vi "eyecat v01 Mc 804 ROB_JS.vi"() -> ()   [LabVIEW 2014]
doc: "This VI is an upgrade from the WIN 1_v4 that implements the ageing subrutine"
uses:
  <vilib>/Utility/file.llb/Write To Spreadsheet File (string).vi
  <vilib>/Utility/file.llb/Read From Spreadsheet File (string).vi
  <vilib>/regexp/Match Regular Expression.xnode
  Controls Win/Control 3.ctl
  <vilib>/Utility/miscctls.llb/LVRowAndColumnTypeDef.ctl
  <vilib>/Platform/TimedLoop/XDataNode/XDataNode.xnode
  <vilib>/Platform/TimedLoop/XDataNode/nitl_modes.ctl
  <vilib>/Platform/TimedLoop/XDataNode/XDNodeRunTimeDep.lvlib
  <vilib>/Platform/TimedLoop/XDataNode/wakeup.ctl
  <vilib>/Platform/TimedLoop/XDataNode/timing_clust.ctl
  Buttons/Numeric control.ctl
  Buttons/String input.ctl
  Buttons/Numeric indicator.ctl
  Buttons/String output.ctl
panel:
  out "MKS 1":i16
  out "MKS 2":i16
  out "output cluster":T2
  out "Full system?":bool
  out "Log interval (seconds)":T1
  in  "Flow rate Age":dbl
  in  "Inlet temp Age":dbl
  out "Stopped?":bool
  in  "Stop Cmd":T1
  out "Connected?":bool
  out "Error":dbl
  out "Iteration Duration":i64
  out "Finished Late? [i-1]":bool
  in  "SO2 ppm":dbl
  out "Furnace temp 1":dbl
  out "stop 2":bool
  in  "Enum 1":i16=1
  in  "Acknowledge":bool
  out "Test number":u16
  out "Flag1":bool=TRUE
  out "EditPos Subc":T3
  out "Flag 2":bool=TRUE
  in  "Tab Control":T4(tab)
  out "Doors Unlocked":bool
  in  "Temperature Limit (°C)":T1=800.0 min=0.0 max=1200.0 step=1.0
  in  "Log Test Button":bool
  in  "File Name":T5
  in  "File Path":path=path "C:/DATA LOG"
  out "Fail":bool
  out "Pass":bool
  in  "Select Test Type":T6(radio)
  out "Standby":bool
  out "Doors Open":bool
  out "Extractor Fan On":bool
  out "Test In Progress":bool
  out "Cool Down":bool
  out "System Alarm":bool
  in  "Execute Leak Test Button":bool
  in  "Stop Test Button":bool
  in  "Start Test Button":bool
  in  "Advanced settings":bool
  out "Lambda 1":dbl
  out "FlowRate":dbl
  out "Tank P":dbl
  out "O2 Rapidox":dbl
  in  "AirB":dbl
  in  "H2O":dbl
  in  "SO2":dbl
  in  "N2":dbl
  in  "CO2":dbl
  in  "NO":dbl
  in  "Air":dbl
  in  "HC":dbl
  in  "CO":dbl
  in  "Output range Lo":dbl=20.0
  in  "Output range Hi":dbl=200.0
  in  "Lambda D":dbl
  in  "Lambda I":dbl
  in  "Lambda P":dbl
  in  "Tank Lo":dbl=7.0
  in  "Tank Hi":dbl=8.0
  in  "Furnace lambda":dbl
  in  "Air Bal Factor":dbl
  in  "Air open loop factor":dbl
  in  "Lambda Setpoint":dbl=1.08
  in  "N2 Age":dbl
  in  "Bed target":dbl=750.0
  in  "Furnace SP WarmUp":dbl=1000.0
  in  "HC Inj Control":dbl
  in  "HC Bal Factor":dbl
  in  "HC Cyc Factor":dbl
  in  "Fan Speed V":dbl
  in  "Air O2 Rap limit":dbl
  in  "Factor Air Baseline":dbl
  in  "SW time":dbl
  in  "Inlet Temperature (°C)":T1=400.0 min=350.0 max=1000.0 step=1.0
  in  "Inlet LAMBDA Rich":T1=0.9 min=0.85 max=0.96 step=0.001
  in  "Inlet LAMBDA Lean":T1=1.2 min=1.02 max=3.0 step=0.001
  in  "Test Stop temperature (°C)":T1=300.0 min=100.0 max=1000.0 step=1.0
  in  "Test Start Temperature (°C)":T1=125.0 min=0.0 max=500.0 step=1.0
  in  "Furnace Ramp Rate (°C/min)":T1=15.0 min=1.0 max=50.0 step=0.1
  in  "NO:CO Ratio":T1=1.1 min=1.0 max=5.0 step=0.1
  in  "Inlet O2 (%)":T1=0.5 min=0.0 max=14.0 step=0.01
  in  "Inlet LAMBDA":T1=1.0 min=0.6 max=3.0 step=0.001
  out "Space Velocity (h-1)":T7
  out "Vol Flow @ STP (l/min)":T7
  in  "Test Flow Rate(g/s)":T1 min=0.0 max=100.0 step=0.01
  out "Sample Volume (litres)":T7
  in  "Number of Samples":T1=1.0 min=1.0 max=6.0 step=1.0
  in  "Sample Diameter (mm)":T1
  out "CO Theory (%)":T7 format="%#_3g"
  out "CO Theory (%)":T7 format="%#_3g"
  out "HC Theory (%)":T7
  in  "Sample Length (mm)":T1 min=0.0 step=0.5
  in  "NO ppm SW":dbl=500.0 caption="NO (ppm)" min=0.0 max=500.0 step=1.0
  in  "NO ppm Loff":T1 caption="NO ppm"
  out "Inlet Temp":dbl
  in  "Delete sCycle":bool
  in  "Load sCycle":bool
  in  "Save sCycle":bool
  in  "Clear subcycle":bool
  in  "Clear Cycle Pattern":bool
  in  "Save Cycle":bool
  in  "Load Cycle":bool
  in  "Delete Cycle":bool
  out "Test Compiled":bool
  in  "Compile Test Button":bool
  in  "Sub-Cycle List":i32(listbox)=1
  in  "Cycle List":i32(listbox)=2
  out "Total Test Duration (hrs)":T8
  in  "Ageing Gas":enum32{"Radio Selection 1", "Radio Selection 2"}(radio)
  in  "Sub-Cycle Pattern":string[][](table) caption="Subcycle pattern"
  in  "Total Number of Cycles":T1=1.0 min=1.0 max=10000.0 step=1.0
  in  "Cycle Pattern":string[][](table)
  in  "Sub-Cycle Name":T5
  in  "Cycle Name":T5
  out "Heat Exchanger Temperatures (°C)":dynamicdata(graph)
  out "Flow Rate (g/s)":dynamicdata(graph)
  out "Sample Temperatures (°C)":dynamicdata(graph)
  out "System Temperatures (°C)":dynamicdata(graph)
  out "HC Concentration (ppm)":dynamicdata(graph)
  out "Lambda":dynamicdata(graph)
  out "M584L Upstream & Downstream":dynamicdata(graph)
  out "NO Concentration (ppm)":dynamicdata(graph)
  in  "Purge System":bool
  in  "Alarm ack":bool
  in  "Clear log":bool
  out "Table":string[][](table)
  out "Soft Alarm":bool
  out "Hard Alarm":bool
  # "Test Type"
  # "Test Commands"
  # "System Indicators"
  # "Leak Test"
  # "Catalyst Specification"
  # "Lightoff Settings"
  # "Furnace Lightoff Settings"
  # "Sweep Settings"
  # "CO/HC Lightoff Settings"
  # "0.96 < lambda < 0.85"
  # "1.02< lambda < 1.6"
  # "350 < Tinlet < 1000"
  # "NO Lightoff Settings"
  # "Flow Specification"
  # "Cycle Compiled"
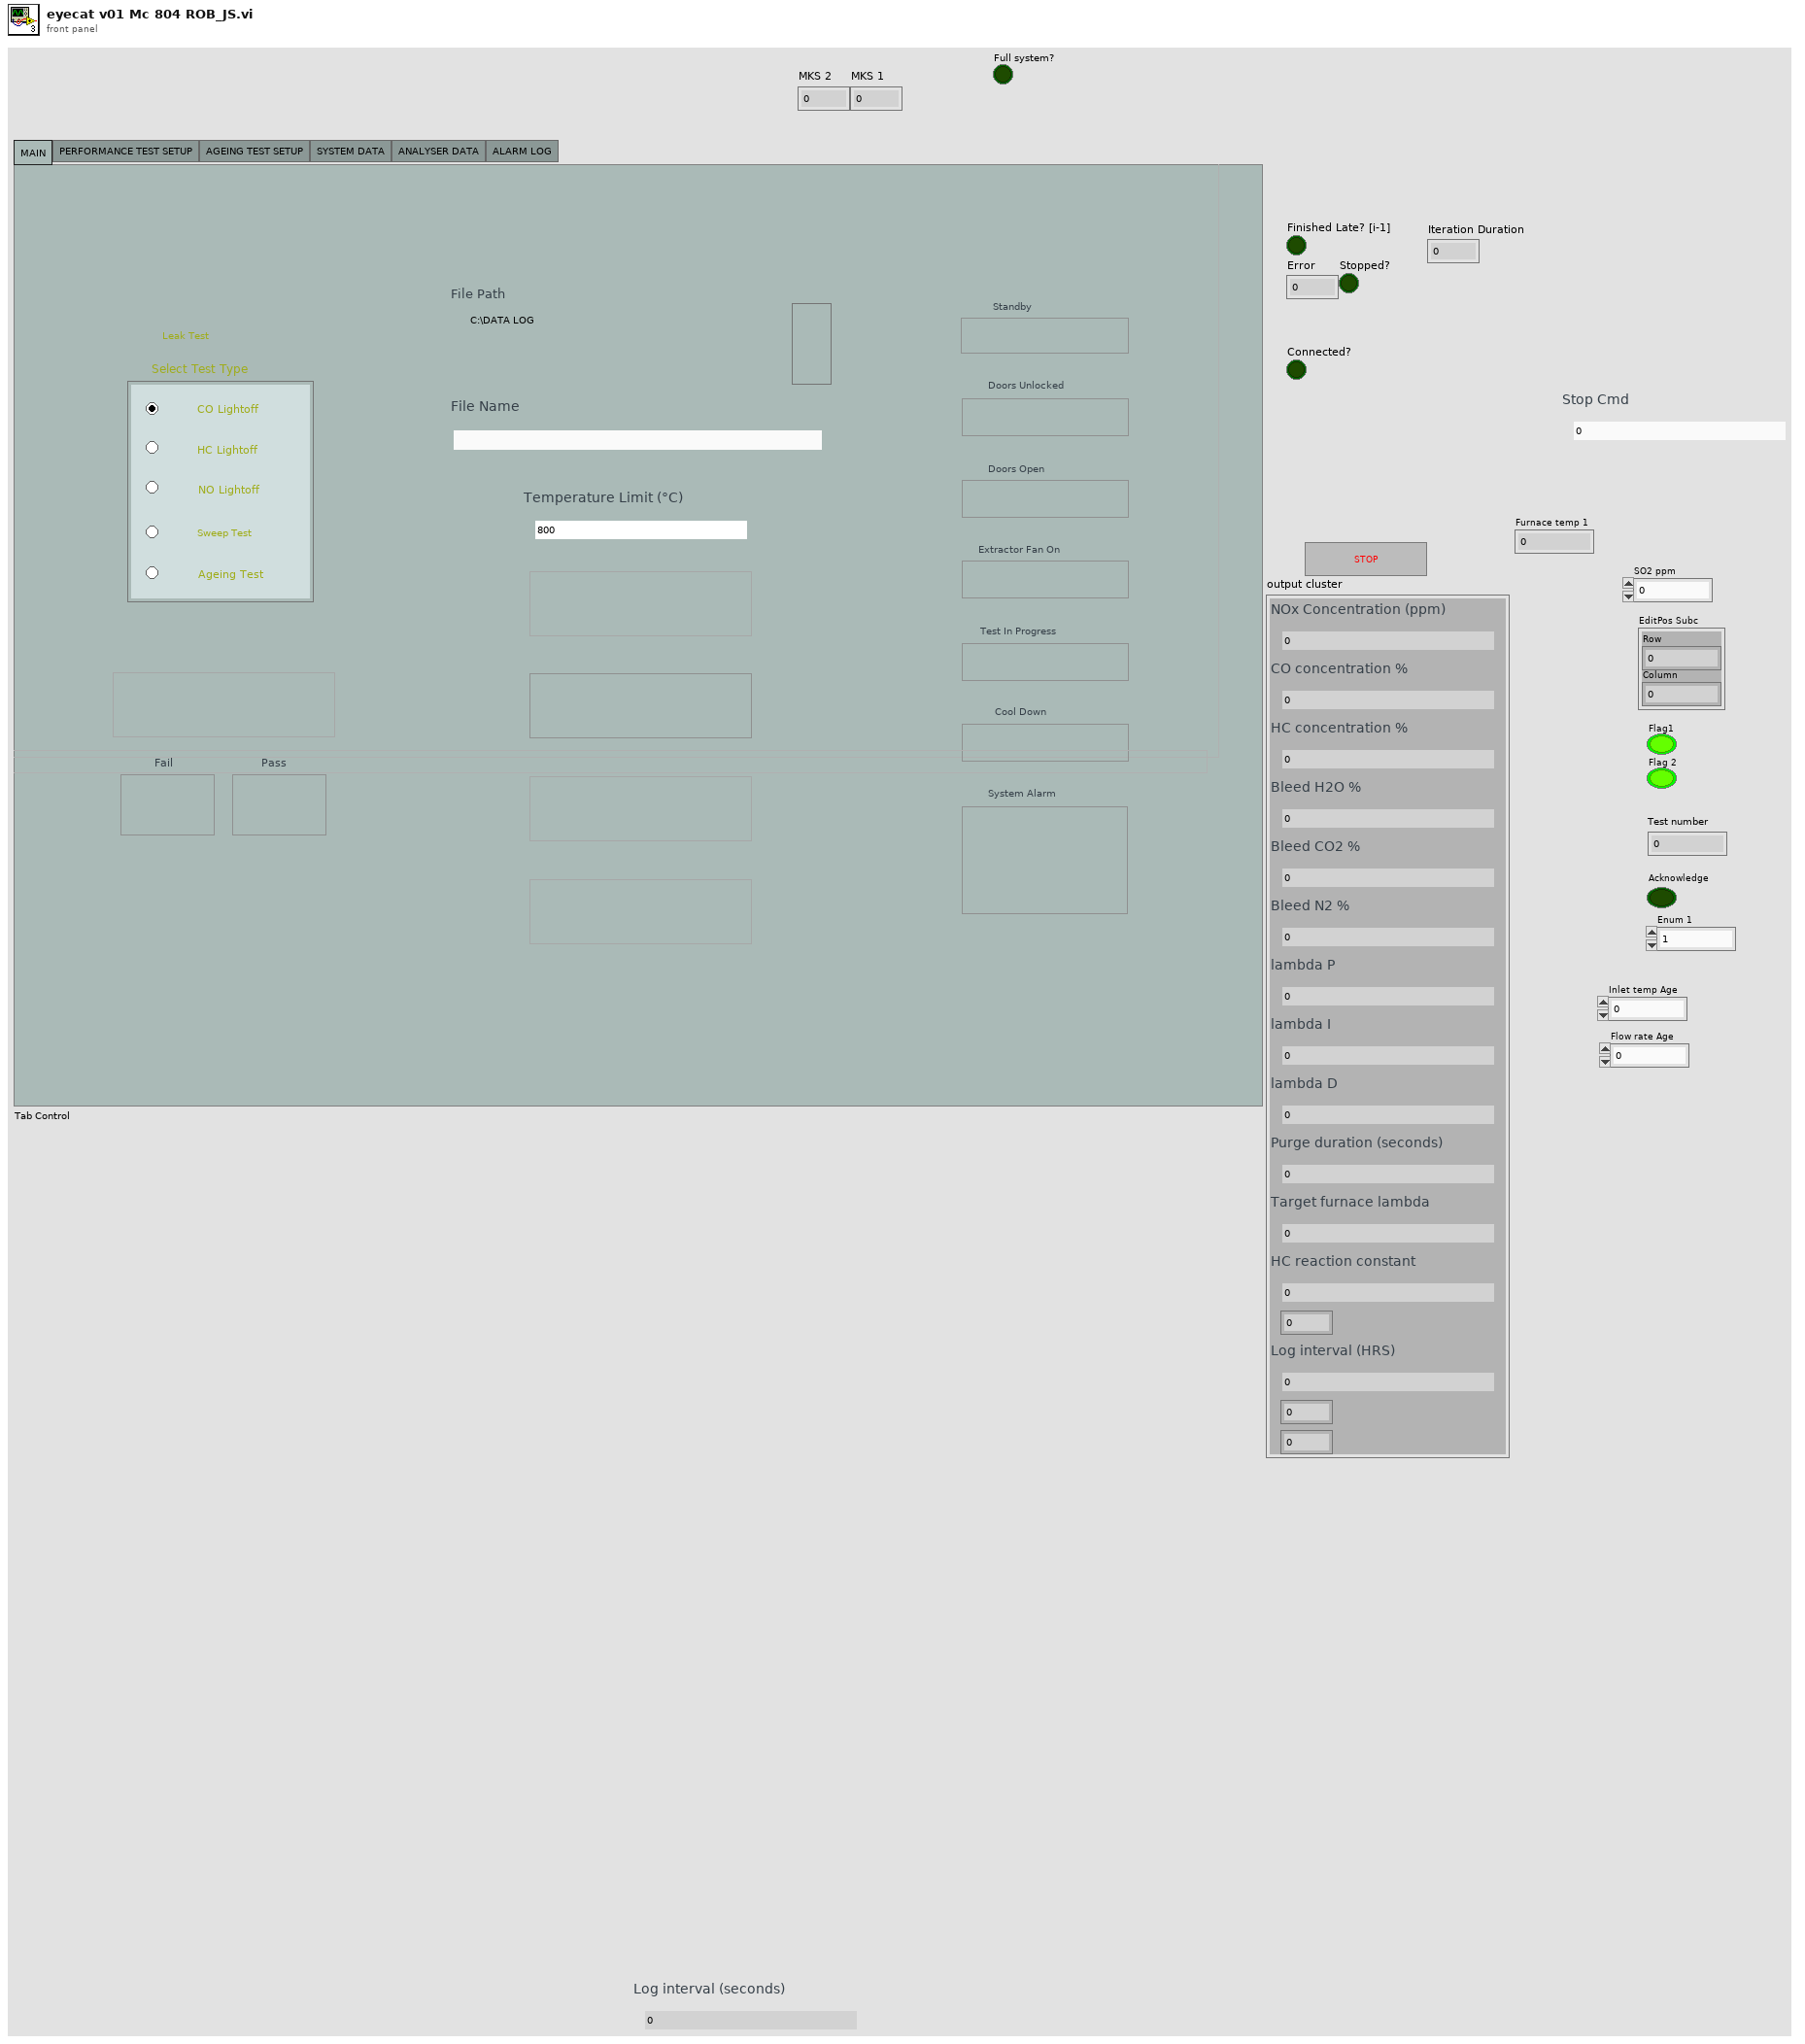
[diagram p1: front panel]
types:
  T1 = typedef "Numeric control.ctl" = dbl
  T2 = cluster{"NOx Concentration (ppm)":T1, "CO concentration %":T1, "HC concentration %":T1, "Bleed H2O %":T1, "Bleed CO2 %":T1, "Bleed N2 %":T1, "lambda P":T1, "lambda I":T1, "lambda D":T1, "Purge duration (seconds)":T1, "Target furnace lambda":T1, "HC reaction constant":T1, i16, "Log interval (HRS)":T1, i16, i16}
  T3 = typedef "LVRowAndColumnTypeDef.ctl" = cluster{"Row":i32, "Column":i32}
  T4 = enum32{"MAIN", "PERFORMANCE TEST SETUP", "AGEING TEST SETUP", "SYSTEM DATA", "ANALYSER DATA", "ALARM LOG"}
  T5 = typedef "String input.ctl" = string
  T6 = enum32{"CO Lightoff", "HC Lightoff", "NO Lightoff", "Sweep Test", "Ageing Test"}
  T7 = typedef "Numeric indicator.ctl" = dbl
  T8 = typedef "String output.ctl" = string
  T9 = typedef "XDNodeRunTimeDep.lvlib/nitl_modes.ctl" = enum32{"No Change", "Process missed periods, maintain original phase", "Discard missed periods, maintain original phase", "Process missed periods, ignore original phase", "Discard missed periods, ignore original phase"}
  T10 = typedef "Control 3.ctl" = enum16{"main", "start test", "save subc", "load subc", "delete subc", "clear table 1", "update list 1", "save cycle", "load cycle", "delete cycle", "clear table 2", "update list 2", "calc HC CO", "Total time calc", "update Cycle pattern ", "load cycle name", "convert to num", "load test array", "check scycle name", "check cycle name", "Multigas connect", "Multigas disconnect"}
  T11 = typedef "XDNodeRunTimeDep.lvlib/timing_clust.ctl" = cluster{"Expected End [f-1]":u64, "Actual End [f-1]":u64, "Finished Late? [f-1]":bool, "Expected End [i-1]":u64, "Actual End [i-1]":u64, "Finished Late? [i-1]":bool, "Expected Start [i]":u64, "Actual Start [i]":u64, "Expected Start [f]":u64, "Actual Start [f]":u64, "Source Name":string, "Structure Name":string, "Period":i64, "Deadline":i64, "Offset":i64, "Start":i64, "Priority":i32, "Timeout":i32, "Mode":T9, "Wakeup Reason":T12, "Error":errorcluster, "Source Type":string, "Secondary Source Type":string, "Global End Time":u64, "Global Start Time":u64, "Frame Duration":u64, "Iteration Duration":u64, "Assigned CPU":i32, "I/O Scan Engine Mode":u32}
  T12 = typedef "XDNodeRunTimeDep.lvlib/wakeup.ctl" = enum32{"Normal", "Aborted", "Asynchronous wakeup", "Timing source error", "Timed loop error", "Timeout"}
  T13 = enum8{"Enabled", "Disabled", "Disabled and Grayed Out"}
  T14 = cluster{"NOx Concentration (ppm)":T1, "CO concentration %":T1, "HC concentration %":T1, "Bleed H2O %":T1, "Bleed CO2 %":T1, "Bleed N2 %":T1, "lambda P":T1, "lambda I":T1, "lambda D":T1, "Purge duration (seconds)":T1, "Target furnace lambda":T1, "HC reaction constant":T1, "Full System?":i16, "Log interval (HRS)":T1}
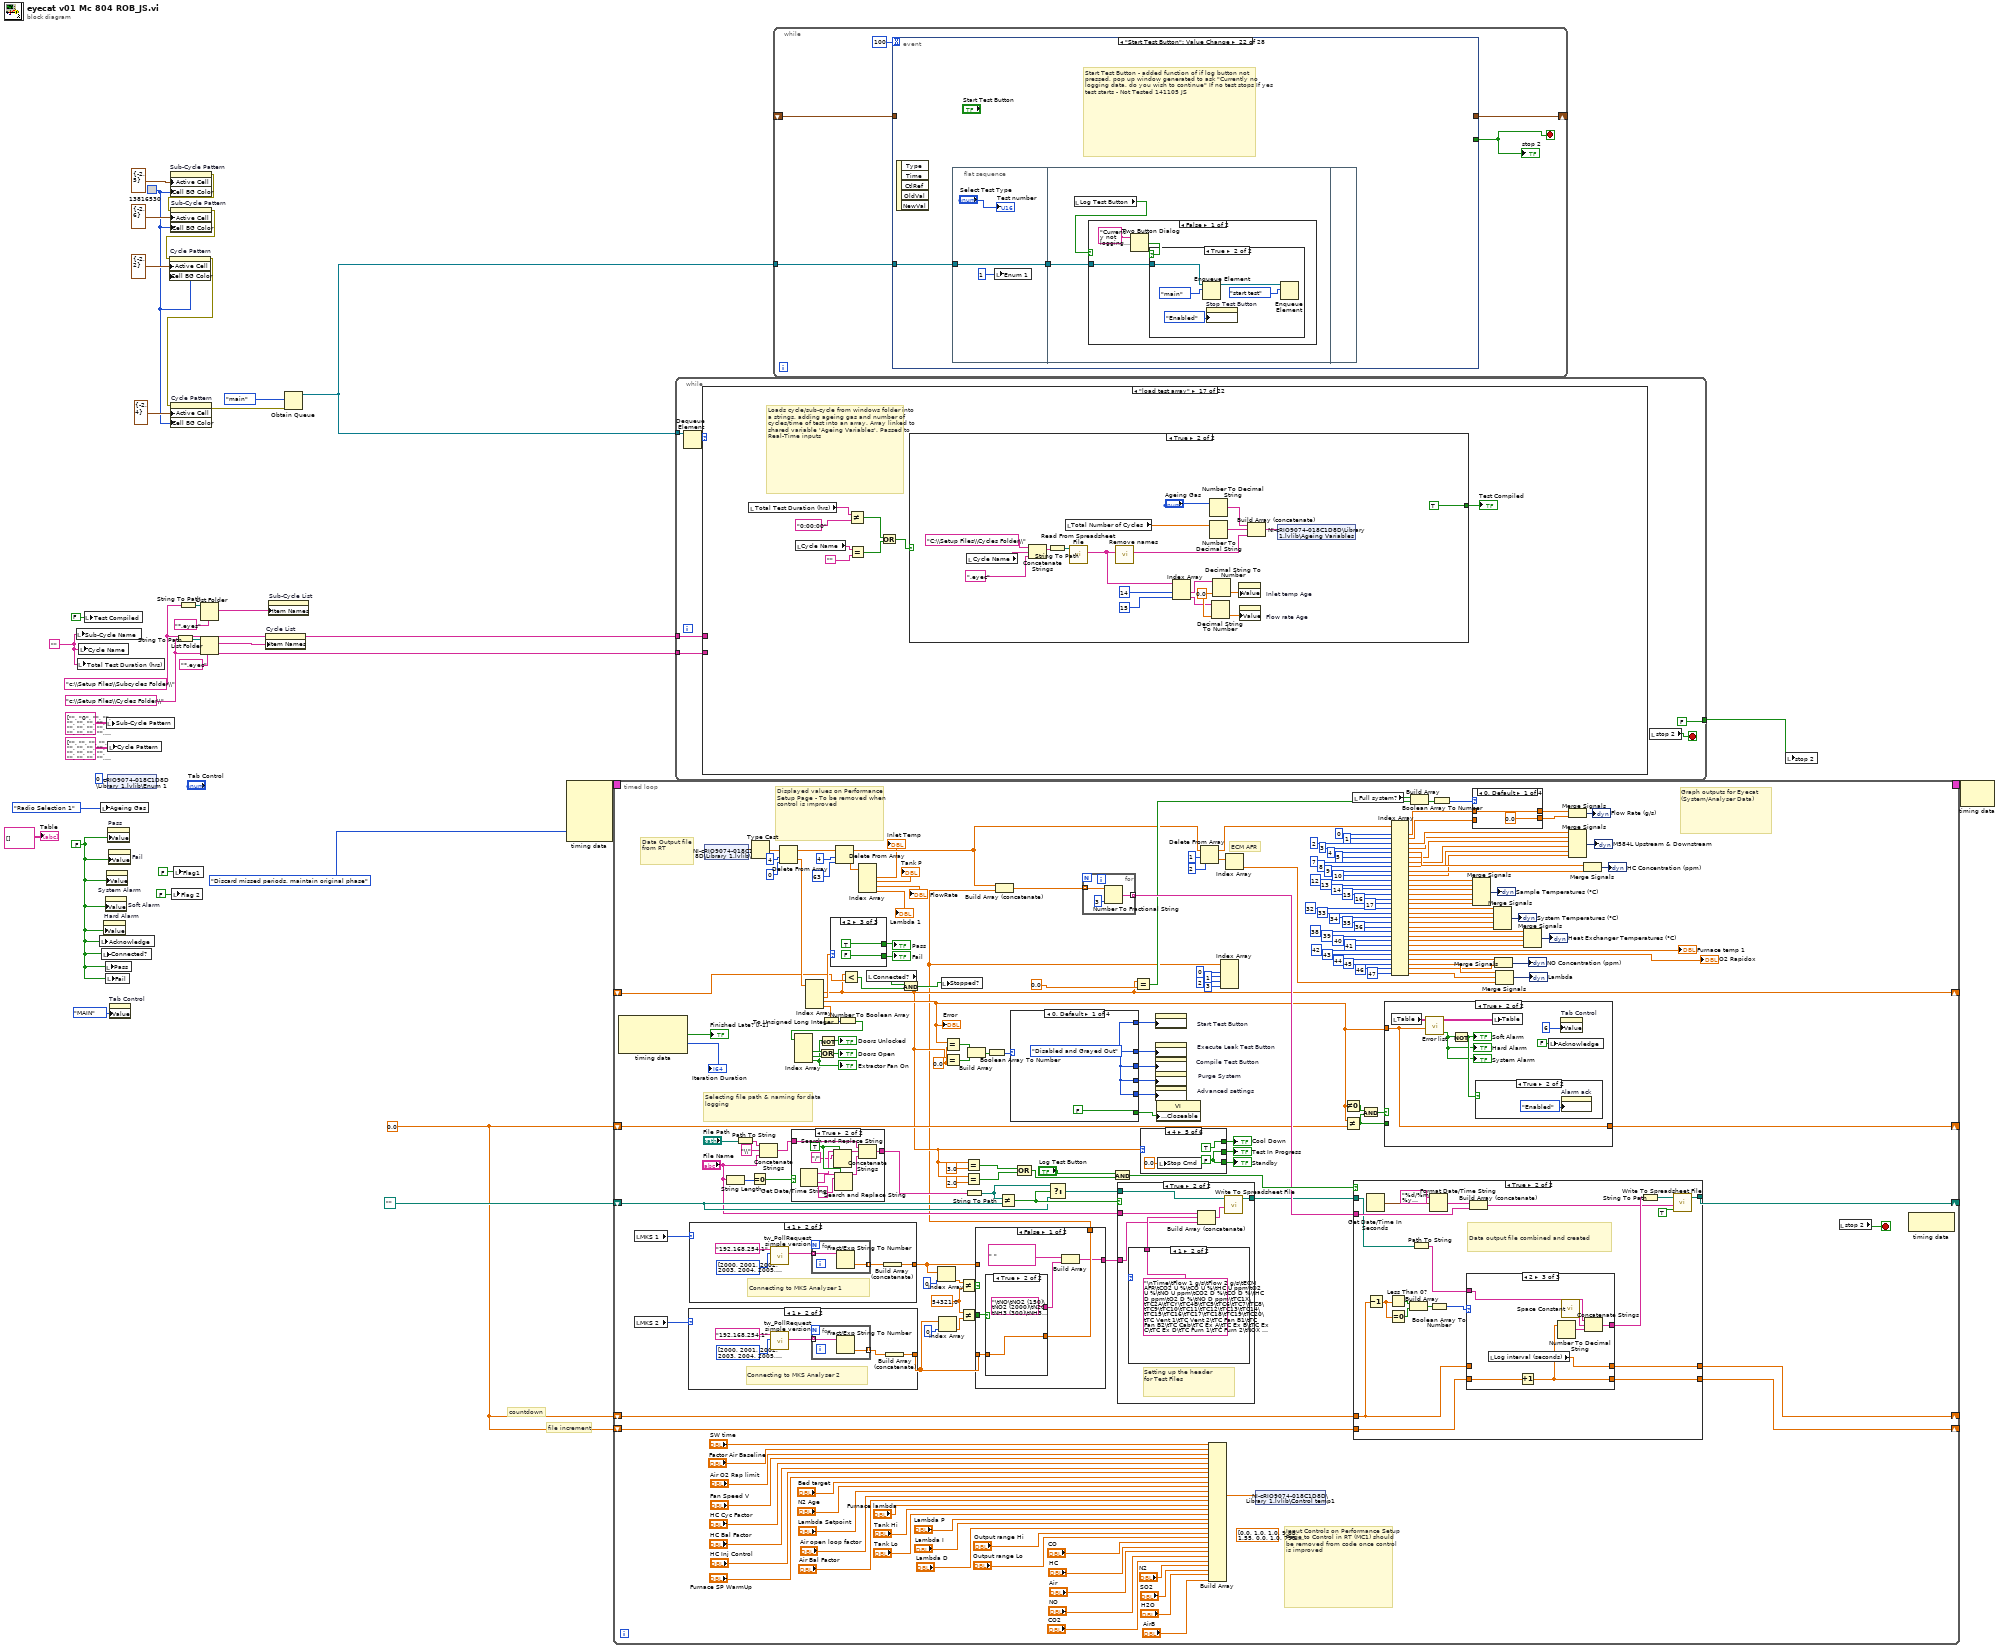
[diagram p0: block diagram]
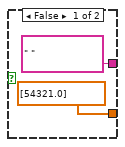
[diagram p2: hidden frame]
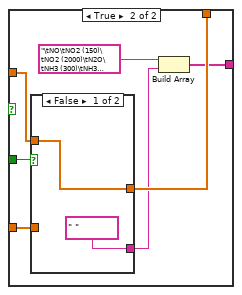
[diagram p3: hidden frame]
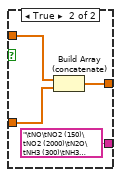
[diagram p4: hidden frame]
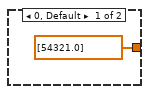
[diagram p5: hidden frame]
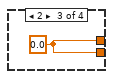
[diagram p7: hidden frame]
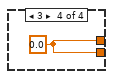
[diagram p8: hidden frame]
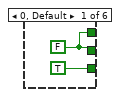
[diagram p10: hidden frame]
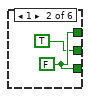
[diagram p11: hidden frame]
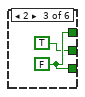
[diagram p12: hidden frame]
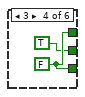
[diagram p13: hidden frame]
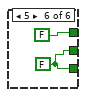
[diagram p14: hidden frame]
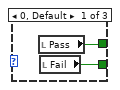
[diagram p15: hidden frame]
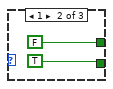
[diagram p16: hidden frame]
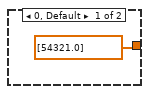
[diagram p17: hidden frame]
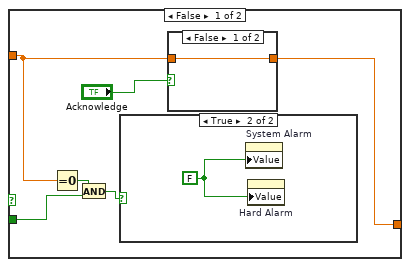
[diagram p18: hidden frame]
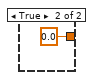
[diagram p19: hidden frame]
diagram:
  w2 = FALSE
  w1 = 0.0 ("y")
  w18 = ""
  w21 = "c:\\Setup Files\\Cycles Folder\\"
  w27 = u32 13816530
  w19 = "c:\\Setup Files\\Subcycles Folder\\"
  # "file increment"
  # "countdown"
  n1 = local write "Sub-Cycle Name"(w18) -> ()
  n2 = local write "Total Test Duration (hrs)"(w18) -> ()
  n3 = local write "Cycle Name"(w18) -> ()
  n4 = local write "Test Compiled"(FALSE ("Cycle Compiled")) -> ()
  n5 = local write "Acknowledge"(w2) -> ()
  n6 = local write "Ageing Gas"(enum32{"Radio Selection 1", "Radio Selection 2"}."Radio Selection 1" ("Ageing Gas")) -> ()
  n7 = local write "Connected?"(w2) -> ()
  n8 = property on="Hard Alarm" class="Bool (strict)"("Value"=w2) -> ()  [unwired: 2 in, 2 out]
  n9 = property on="Soft Alarm" class="Bool (strict)"("Value"=w2) -> ()  [unwired: 2 in, 2 out]
  n10 = local write "Pass"(w2) -> ()
  n11 = local write "Fail"(w2) -> ()
  n12 = local write "Sub-Cycle Pattern"(string[][] [["", "0", "", "", "", "", "", "", "", "", "", "", ""], ["", "", "", "", "", "", "", "", "", "", "", "", ""], ["", "", "", "", "", "", "", "", "", "", "", "", ""], ["", "", "", "", "", "", "", "", "", "", "", "", ""], ["", "", "", "", "", "", "", "", "", "", "", "", ""], ["", "", "", "", "", "", "", "", "", "", "", "", ""], ["", "", "", "", "", "", "", "", "", "", "", "", ""], ["", "", "", "", "", "", "", "", "", "", "", "", ""], ["", "", "", "", "", "", "", "", "", "", "", "", ""], ["", "", "", "", "", "", "", "", "", "", "", "", ""], ["", "", "", "", "", "", "", "", "", "", "", "", ""], ["", "", "", "", "", "", "", "", "", "", "", "", ""], ["", "", "", "", "", "", "", "", "", "", "", "", ""], ["", "", "", "", "", "", "", "", "", "", "", "", ""], ["", "", "", "", "", "", "", "", "", "", "", "", ""], ["", "", "", "", "", "", "", "", "", "", "", "", ""], ["", "", "", "", "", "", "", "", "", "", "", "", ""], ["", "", "", "", "", "", "", "", "", "", "", "", ""], ["", "", "", "", "", "", "", "", "", "", "", "", ""], ["", "", "", "", "", "", "", "", "", "", "", "", ""], ["", "", "", "", "", "", "", "", "", "", "", "", ""], ["", "", "", "", "", "", "", "", "", "", "", "", ""], ["", "", "", "", "", "", "", "", "", "", "", "", ""], ["", "", "", "", "", "", "", "", "", "", "", "", ""], ["", "", "", "", "", "", "", "", "", "", "", "", ""], ["", "", "", "", "", "", "", "", "", "", "", "", ""], ["", "", "", "", "", "", "", "", "", "", "", "", ""], ["", "", "", "", "", "", "", "", "", "", "", "", ""], ["", "", "", "", "", "", "", "", "", "", "", "", ""], ["", "", "", "", "", "", "", "", "", "", "", "", ""], ["", "", "", "", "", "", "", "", "", "", "", "", ""]]) -> ()
  n13 = property on="System Alarm" class="Bool (strict)"("Value"=w2) -> ()  [unwired: 2 in, 2 out]
  n14 = local write "Cycle Pattern"(string[][] [["", "", "", "", ""], ["", "", "", "", ""], ["", "", "", "", ""], ["", "", "", "", ""], ["", "", "", "", ""], ["", "", "", "", ""], ["", "", "", "", ""], ["", "", "", "", ""], ["", "", "", "", ""], ["", "", "", "", ""], ["", "", "", "", ""], ["", "", "", "", ""], ["", "", "", "", ""], ["", "", "", "", ""], ["", "", "", "", ""], ["", "", "", "", ""], ["", "", "", "", ""], ["", "", "", "", ""], ["", "", "", "", ""], ["", "", "", "", ""], ["", "", "", "", ""], ["", "", "", "", ""], ["", "", "", "", ""], ["", "", "", "", ""], ["", "", "", "", ""], ["", "", "", "", ""], ["", "", "", "", ""], ["", "", "", "", ""], ["", "", "", "", ""], ["", "", "", "", ""], ["", "", "", "", ""]]) -> ()
  n15 = shared-variable "NI-cRIO9074-018C1D8D\\Library 1.lvlib\\Enum 1"(u16 0 ("Enum 1")) -> ()  [unwired: 1 in, 1 out]
  n16 = property on="Pass" class="Bool (strict)"("Value"=w2) -> ()  [unwired: 2 in, 2 out]
  n17 = property on="Fail" class="Bool (strict)"("Value"=w2) -> ()  [unwired: 2 in, 2 out]
  n18 = property on="Tab Control" class="TabCtl (strict)"("Value"=T4."MAIN" ("Tab Control")) -> ()  [unwired: 2 in, 2 out]
  n19 = property on="Sub-Cycle Pattern" class="Tbl (strict)"("Active Cell"=T3 {"Row"=-2, "Column"=5} ("Active Cell:Active Cell"), "Cell BG Color"=w27) -> (error out=w32:errorcluster)  [unwired: 2 in, 1 out]
  n20 = property on="Sub-Cycle Pattern" class="Tbl (strict)"(error in=w32, "Active Cell"=T3 {"Row"=-2, "Column"=6} ("Active Cell:Active Cell"), "Cell BG Color"=w27) -> (error out=w31:errorcluster)  [unwired: 1 in, 1 out]
  n21 = property on="Cycle Pattern" class="Tbl (strict)"(error in=w31, "Active Cell"=T3 {"Row"=-2, "Column"=2} ("Active Cell:Active Cell"), "Cell BG Color"=w27) -> (error out=w29:errorcluster)  [unwired: 1 in, 1 out]
  n22 = property on="Cycle Pattern" class="Tbl (strict)"(error in=w29, "Active Cell"=T3 {"Row"=-2, "Column"=4} ("Active Cell:Active Cell"), "Cell BG Color"=w27) -> (error out=w26:errorcluster)  [unwired: 1 in, 1 out]
  n23 = local write "Flag 2"(FALSE) -> ()
  n24 = local write "Flag1"(FALSE) -> ()
  n25 = String To Path(string=w21) -> (path=w22:path)
  n26 = String To Path(string=w19) -> (path=w24:path)
  n27 = List Folder(path=w22, pattern="*.eyec") -> (filenames=w23:string[])  [unwired: 2 in, 3 out]
  n28 = List Folder(path=w24, pattern="*.eyes") -> (filenames=w25:string[])  [unwired: 2 in, 3 out]
  n29 = property on="Cycle List" class="LstBox (strict)"("Item Names"=w23) -> ()  [unwired: 2 in, 2 out]
  n30 = property on="Sub-Cycle List" class="LstBox (strict)"("Item Names"=w25) -> ()  [unwired: 2 in, 2 out]
  n31 = Obtain Queue(element data type=Control_3."main" ("Enum"), error in (no error)=w26) -> (queue out=w35:refnum<queue>)  [unwired: 3 in, 2 out]
  n32 = node-c288(nitl_modes."Discard missed periods, maintain original phase" ("Mode")) -> (w7:T11)  [unwired: 4 in]
  n33 = timed-loop {
    timing: w7 -> [_]
    timing-out: [_] -> w6
    shift-right: [w217] -> _
    shift-left: path "" -> [w219]
    shift-right: [w169] -> _
    shift-left: w1 -> [w218]
    shift-right: [w54] -> _
    shift-left: _ -> [w182]
    shift-right: [w159] -> _
    shift-left: w1 -> [w51]
    shift-right: [w160] -> _
    shift-left: w1 -> [w162]
    stop <- w216 stop-if-true
    w38 = 54321.0 ("y")
    (unwired) dbl[] [0.0, 1.0, 1.0, 9.85, 1.55, 0.0, 1.0, 799.0, 1000.0, 0.0, 1.02, 1.35, 0.0, 1.02, 8.0, 7.0, 40.0, 0.0, 0.0, 20.0, 60.0, 0.0, 1.0, 0.0, 0.0, 0.0, 60.0, 0.0, 0.0, 0.0] ("appended array")
    w199 = 0.0 ("y")
    # "Selecting file path & naming for data logging"
    # "Data Output file from RT"
    # "Displayed values on Performance Setup Page - To be removed when control is improved"
    # "Input Controls on Performance Setup Page to Control in RT (MC1) should be removed from code once control is improved"
    # "Graph outputs for Eyecat (System/Analyser Data)"
    # "ECM AFR"
    n34 = node-c288() -> (→"Finished Late? [i-1]":bool, →"Iteration Duration":i64)  [unwired: 1 in, 1 out]
    n35 = local read "MKS 1"() -> (w205:i16)
    n36 = local read "MKS 2"() -> (w50:i16)
    n37 = case shown="1" w50 {
      tunnel: [dbl[] [54321.0] w275] -> w44
      frame 0, Default {
      }
      frame 1 {
        # "Connecting to MKS Analyser 2"
        n38 = call "tw_PollRequest simple version.vi"("EVID list"=i32[] [2000, 2001, 2002, 2003, 2004, 2005, 2006, 2007, 2008, 2009, 2010, 2011, 2012, 2013, 2014], "IP_ADD [127.0.0.1]"="192.168.254.1") -> ("values out"=w273:string[])  [unwired: 7 in, 2 out]
        n39 = for {
          tunnel: [w277] -> w271 mode=indexing
          tunnel: w273 -> [w276] mode=indexing
          n40 = Fract/Exp String To Number(string=w276) -> (number=w277:dbl)  [unwired: 3 in, 1 out]
        }
        n41 = Build Array (concatenate)(w271) -> (w275:dbl[])
      }
    }
    n42 = case shown="1" w205 {
      tunnel: [dbl[] [54321.0] w314] -> w46
      frame 0, Default {
      }
      frame 1 {
        # "Connecting to MKS Analyser 1"
        n43 = call "tw_PollRequest simple version.vi"("EVID list"=i32[] [2000, 2001, 2002, 2003, 2004, 2005, 2006, 2007, 2008, 2009, 2010, 2011, 2012, 2013, 2014], "IP_ADD [127.0.0.1]"="192.168.254.1") -> ("values out"=w317:string[])  [unwired: 7 in, 2 out]
        n44 = for {
          tunnel: [w320] -> w315 mode=indexing
          tunnel: w317 -> [w319] mode=indexing
          n45 = Fract/Exp String To Number(string=w319) -> (number=w320:dbl)  [unwired: 3 in, 1 out]
        }
        n46 = Build Array (concatenate)(w315) -> (w314:dbl[])
      }
    }
    n47 = shared-variable "NI-cRIO9074-018C1D8D\\Library 1.lvlib\\DATA"() -> (w215:dbl[])  [unwired: 1 in, 1 out]
    n48 = String Length(string="File Name") -> (length=w173:i32)
    n49 = Path To String(path="File Path") -> (string=w175:string)
    n50 = Equal To 0?(x=w173) -> (x = 0?=w172:bool)
    n51 = Type Cast(type=w215, x=w215) -> (*(type *) &x=w227:dbl[])
    n52 = Concatenate Strings(w175, "\\" ("string"), "File Name") -> (w171:string)
    n53 = Delete From Array(array=w227, length=4, index=0) -> (deleted portion=w224:dbl[], array with subset deleted=w64:dbl[])
    n54 = case shown="True" w172 {
      tunnel: [w284 w292] -> w161
      tunnel: w171 -> [w284 w293]
      frame False {
      }
      frame True {
        w290 = TRUE ("replace all? (F)")
        n55 = Get Date/Time String() -> (date string=w288:string, time string=w289:string)  [unwired: 3 in]
        n56 = Search and Replace String(replace all?=w290, input string=w288, search string="/") -> (result string=w291:string)  [unwired: 5 in, 3 out]
        n57 = Search and Replace String(replace all?=w290, input string=w289, search string=":") -> (result string=w285:string)  [unwired: 5 in, 3 out]
        n58 = Concatenate Strings(w293, w291, w285) -> (w292:string)
      }
    }
    n59 = Index Array(array=w224) -> (element #1=w54:dbl, element #2=w188:dbl, element #3=w189:dbl, element #4=w181:dbl)  [unwired: 4 in]
    "Error" <- w189
    n60 = To Unsigned Long Integer(number=w181) -> (unsigned 32bit integer=w180:u32)
    n61 = case shown="2" w188 {
      tunnel: [w307 TRUE FALSE] -> w187
      tunnel: [w308 FALSE TRUE] -> w186
      frame 0, Default {
        n62 = local read "Pass"() -> (w308:bool)
        n63 = local read "Fail"() -> (w307:bool)
      }
      frame 1 {
      }
      frame 2 {
      }
    }
    "Pass" <- w186
    "Fail" <- w187
    n64 = Delete From Array(array=w64, length=4, index=63) -> (deleted portion=w60:dbl[], array with subset deleted=w63:dbl[])
    n65 = Number To Boolean Array(number=w180) -> (Boolean array=w204:bool[])
    n66 = Index Array(array=w204) -> (element #2=w202:bool, element #3=w201:bool, element #4=w177:bool)  [unwired: 4 in, 1 out]
    "Extractor Fan On" <- w177
    n67 = Or(x=w202, y=w201) -> (x .or. y?=→"Doors Open":bool)
    n68 = Not(x=w177) -> (.not. x?=→"Doors Unlocked":bool)
    n69 = Less?(x=w54, y=w182) -> (x < y?=w179:bool)
    n70 = Index Array(array=w60) -> (element #1=→"Inlet Temp":dbl, element #2=→"Tank P":dbl, element #3=→"FlowRate":dbl, element #4=→"Lambda 1":dbl)  [unwired: 4 in]
    n71 = local read "Connected?"() -> (w178:bool)
    n72 = And(x=w178, y=w179) -> (x .and. y?=w168:bool)
    n73 = Index Array(array=w46, index=0) -> (element=w42:dbl)
    n74 = Index Array(array=w44, index=0) -> (element=w40:dbl)
    n75 = local write "Stopped?"(w168) -> ()
    n76 = Equal?(x=w189, y=w199) -> (x = y?=w197:bool)
    n77 = Equal?(x=w54, y=w199) -> (x = y?=w196:bool)
    n78 = Not Equal?(x=w42, y=w38) -> (x != y?=w41:bool)
    n79 = Not Equal?(x=w38, y=w40) -> (x != y?=w39:bool)
    n80 = Equal?(x=w54, y=3.0) -> (x = y?=w102:bool)
    n81 = Equal?(x=w54, y=2.0) -> (x = y?=w52:bool)
    n82 = String To Path(string=w161) -> (path=w170:path)
    n83 = Build Array(w197, w196) -> (w195:bool[])
    n84 = case shown="False" w41 {
      tunnel: [w252 w263] -> w47
      tunnel: w44 -> [w251 w262]
      tunnel: w46 -> [_ w261]
      tunnel: w39 -> [w250 w260]
      tunnel: [w249 w257] -> w37
      frame False {
        n85 = case shown="True" w250 {
          tunnel: [dbl[] [54321.0] w256] -> w252
          tunnel: w251 -> [_ w256]
          tunnel: [" " ("Heading string 2") "\tNO\tNO2 (150)\tNO2 (2000)\tN2O\tNH3 (300)\tNH3 (3000)\tHNCO (400)\tH2O\tCO2\tCO (500)\tCO (1)\tCH4 (250)\tCH4 (3000)\tNOxP\tPropane" ("Heading string 2")] -> w247
          frame False {
          }
          frame True {
          }
        }
        n86 = Build Array(" " ("Heading string 2"), w247) -> (w249:string[])
      }
      frame True {
        n87 = case shown="False" w260 {
          tunnel: [w265 w269] -> w263
          tunnel: w262 -> [_ w268]
          tunnel: w261 -> [w265 w267]
          tunnel: [" " ("Heading string 2") "\tNO\tNO2 (150)\tNO2 (2000)\tN2O\tNH3 (300)\tNH3 (3000)\tHNCO (400)\tH2O\tCO2\tCO (500)\tCO (1)\tCH4 (250)\tCH4 (3000)\tNOxP\tPropane" ("Heading string 2")] -> w258
          frame False {
          }
          frame True {
            n88 = Build Array (concatenate)(w267, w268) -> (w269:dbl[])
          }
        }
        n89 = Build Array("\tNO\tNO2 (150)\tNO2 (2000)\tN2O\tNH3 (300)\tNH3 (3000)\tHNCO (400)\tH2O\tCO2\tCO (500)\tCO (1)\tCH4 (250)\tCH4 (3000)\tNOxP\tPropane" ("Heading string 2"), w258) -> (w257:string[])
      }
    }
    n90 = Boolean Array To Number(Boolean array=w195) -> (number=w194:u32)
    n91 = Build Array (concatenate)(w63, w47) -> (w220:dbl[])
    n92 = Not Equal?(x=w170, y=w219) -> (x != y?=w229:bool)
    n93 = case shown="0, Default" w194 {
      tunnel: [w339 w341 w343 w346] -> w198
      tunnel: [w339 w341 w343 w346] -> w193
      tunnel: [w339 w341 w343 w346] -> w192
      tunnel: [w339 w341 T13."Enabled" ("Disabled") w346] -> w191
      tunnel: [w339 w341 w343 w346] -> w190
      tunnel: [FALSE FALSE FALSE TRUE] -> w167
      frame 0, Default {
        w339 = T13."Disabled and Grayed Out" ("Disabled")
      }
      frame 1 {
        (unwired) T13."Enabled" ("Disabled")
        w341 = T13."Disabled and Grayed Out" ("Disabled")
      }
      frame 2 {
        w343 = T13."Disabled and Grayed Out" ("Disabled")
      }
      frame 3 {
        w346 = T13."Enabled" ("Disabled")
        (unwired) T13."Disabled and Grayed Out" ("Disabled")
      }
    }
    n94 = Compound Arithmetic op=OR(w102, w52) -> (w101:bool)
    n95 = Select(t=w170, s=w229, f=w219) -> (s? t:f=w230:path)
    n96 = for {
      tunnel: w220 -> [w357] mode=indexing
      tunnel: [w356] -> w231 mode=indexing
      n97 = Number To Fractional String(number=w357, precision (6)=i16 3) -> (F-format string=w356:string)  [unwired: 2 in]
    }
    n98 = And(x="Log Test Button", y=w101) -> (x .and. y?=w246:bool)
    n99 = case shown="True" w229 {
      tunnel: w230 -> [w347 w353]
      tunnel: [w347 w352] -> w228
      tunnel: "File Name" -> [_ w350]
      tunnel: w37 -> [_ w348]
      frame False {
      }
      frame True {
        # "Setting up the header\nfor Test Files"
        n100 = case shown="1" {
          selector: _ -> [_ _]
          tunnel: ["\nTime\tFlow 1 g/s\tFlow 2 g/s\tECM AFR\tCO2 U %\tCO U %\tHC U ppm\tO2 U %\tNO U ppm\tCO2 D %\tCO D %\tHC D ppm\tO2 D %\tNO D ppm\tTC1X\tTC2A\tTCY\tTC4B\tTC5\tTC6\tTC7\tTC8\tTC9\tTC10\tTC11\tTC12\tTC13\tTC14\tTC15\tTC16\tTC17\tTC18\tTC19\tTC20\tNOX 1 ppm\tNLambda 1\tNOX 2 ppm\tNLambda 2\tEGO 1\tEGO 2\t" ("Heading string 2") "\nTime\tFlow 1 g/s\tFlow 2 g/s\tECM AFR\tCO2 U %\tCO U %\tHC U ppm\tO2 U %\tNO U ppm\tCO2 D %\tCO D %\tHC D ppm\tO2 D %\tNO D ppm\tTC1X\tTC2A\tTCY\tTC4B\tTC5\tTC6\tTC7\tTC8\tTC9\tTC10\tTC11\tTC12\tTC13\tTC14\tTC15\tTC16\tTC17\tTC18\tTC19\tTC20\tTC Vent 1\tTC Vent 2\tTC Fan B1\tTC Fan B2\tTC Cab\tTC Ex A\tTC Ex B\tTC Ex C\tTC Ex D\tTC Furn 1\tTC Furn 2\tNOX 1 ppm\tNLambda 1\tNOX 2 ppm\tNLambda 2\tEGO 1\tEGO 2\tEGO 3\tEGO 4\tCO2 U %\tCO U %\tHC U ppm\tO2 U %\tNO U ppm\tCO2 D %\tCO D %\tHC D ppm\tO2 D %\tNO D ppm\r\n" ("Heading string 2")] -> w349
          frame 0, Default {
          }
          frame 1 {
          }
        }
        n101 = Build Array (concatenate)(w350, w349, w348) -> (w351:T5[])
        n102 = call-poly <vilib>:"Write To Spreadsheet File.vi"("1D data"=w351, "file path (dialog if empty)"=w353) -> ("new file path (Not A Path if cancelled)"=w352:path)  [unwired: 6 in]
      }
    }
    n103 = Equal?(x=w54, y=0.0) -> (x = y?=w156:bool)
    n104 = case shown="4" w54 {
      tunnel: [w294 w297 w299 w301 TRUE FALSE] -> w185
      tunnel: [w294 TRUE TRUE TRUE w303 w305] -> w184
      tunnel: [TRUE w297 w299 w301 w303 w305] -> w183
      frame 0, Default {
        w294 = FALSE
      }
      frame 1 {
        w297 = FALSE
      }
      frame 2 {
        w299 = FALSE
      }
      frame 3 {
        w301 = FALSE
      }
      frame 4 {
        w303 = FALSE
        n105 = local write "Stop Cmd"(T1 0.0 ("Stop Cmd")) -> ()
      }
      frame 5 {
        w305 = FALSE
      }
    }
    "Cool Down" <- w185
    "Test In Progress" <- w184
    "Standby" <- w183
    n106 = property on="Start Test Button" class="Bool"("DisabledEnum"=w198) -> ()  [unwired: 2 in, 2 out]
    n107 = property on="Execute Leak Test Button" class="Bool"("DisabledEnum"=w193) -> ()  [unwired: 2 in, 2 out]
    n108 = property on="Compile Test Button" class="Bool"("DisabledEnum"=w192) -> ()  [unwired: 2 in, 2 out]
    n109 = property on="Purge System" class="Bool"("DisabledEnum"=w191) -> ()  [unwired: 2 in, 2 out]
    n110 = property on="Advanced settings" class="Bool"("DisabledEnum"=w190) -> ()  [unwired: 2 in, 2 out]
    n111 = property class="VI"("Front Panel.Closeable"=w167) -> ()  [unwired: 2 in, 2 out]
    n112 = Delete From Array(array=w63, length=1, index=2) -> (deleted portion=w98:dbl[], array with subset deleted=w96:dbl[])
    n113 = Build Array("SW time", "Factor Air Baseline", "Air O2 Rap limit", "Fan Speed V", "HC Cyc Factor", "HC Bal Factor", "HC Inj Control", "Furnace SP WarmUp", "Bed target", "N2 Age", "Lambda Setpoint", "Air open loop factor", "Air Bal Factor", "Furnace lambda", "Tank Hi", "Tank Lo", "Lambda P", "Lambda I", "Lambda D", "Output range Hi", "Output range Lo", "CO", "HC", "Air", "NO", "CO2", "N2", "SO2", "H2O", "AirB") -> (w89:dbl[])
    n114 = Index Array(array=w47, index #1=0 ("index"), index #2=1 ("index"), index #3=2 ("index"), index #4=3 ("index")) -> ()  [unwired: 4 out]
    n115 = Index Array(array=w98) -> (element=w97:dbl)  [unwired: 1 in]
    n116 = shared-variable "NI-cRIO9074-018C1D8D\\Library 1.lvlib\\Control temp1"(w89) -> ()  [unwired: 1 in, 1 out]
    n117 = Not Equal To 0?(x=w189) -> (x != 0?=w222:bool)
    n118 = Not Equal?(x=w189, y=w218) -> (x != y?=w221:bool)
    n119 = local read "Full system?"() -> (w157:bool)
    n120 = case shown="True" w246 {
      tunnel: w228 -> [w361 w369]
      tunnel: [w361 w381] -> w217
      tunnel: w231 -> [_ w377]
      tunnel: w51 -> [_ w370]
      tunnel: w162 -> [w360 w365]
      tunnel: [w360 w367] -> w160
      tunnel: [w359 w366] -> w159
      frame False {
        n121 = local read "Log interval (seconds)"() -> (w359:T1)
      }
      frame True {
        # "Data output file combined and created"
        n122 = Get Date/Time In Seconds() -> (seconds since 1Jan1904=w378:timestamp)
        n123 = Decrement(x=w370) -> (x-1=w371:T1)
        n124 = Less Than 0?(x=w371) -> (x < 0?=w372:bool)
        n125 = Equal To 0?(x=w371) -> (x = 0?=w373:bool)
        n126 = Build Array(w372, w373) -> (w374:bool[])
        n127 = Path To String(path=w369) -> (string=w364:string)
        n128 = Format Date/Time String(time format string (%c)="%d/%m/%y %H:%M:%S", seconds (now)=w378) -> (date/time string=w379:string)  [unwired: 1 in]
        n129 = Boolean Array To Number(Boolean array=w374) -> (number=w375:u32)
        n130 = case shown="2" w375 {
          tunnel: w370 -> [w388 w389 _]
          tunnel: [w387 w389 w392] -> w366
          tunnel: w364 -> [w386 w391 w395]
          tunnel: [w383 w391 w393] -> w368
          tunnel: [w382 w390 w394] -> w367
          tunnel: w365 -> [w382 w390 w398]
          frame 0, Default {
            n131 = Number To Decimal String(number=w382) -> (decimal integer string=w384:string)  [unwired: 1 in]
            n132 = call <vilib>:"Space Constant.vi"() -> ("String"=w385:string)
            n133 = Decrement(x=w388) -> (x-1=w387:T1)
            n134 = Concatenate Strings(w386, w385, w384) -> (w383:string)
          }
          frame 1 {
          }
          frame 2 {
            n135 = local read "Log interval (seconds)"() -> (w392:T1)
            n136 = Increment(x=w398) -> (x+1=w394:dbl)
            n137 = Number To Decimal String(number=w394) -> (decimal integer string=w396:string)  [unwired: 1 in]
            n138 = call <vilib>:"Space Constant.vi"() -> ("String"=w397:string)
            n139 = Concatenate Strings(w395, w397, w396) -> (w393:string)
          }
        }
        n140 = Build Array (concatenate)(w379, w377) -> (w363:string[])
        n141 = String To Path(string=w368) -> (path=w362:path)
        n142 = call-poly <vilib>:"Write To Spreadsheet File.vi"("append to file? (new file:F)"=TRUE, "1D data"=w363, "file path (dialog if empty)"=w362) -> ("new file path (Not A Path if cancelled)"=w381:path)  [unwired: 5 in]
      }
    }
    n143 = And(x=w222, y=w221) -> (x .and. y?=w223:bool)
    n144 = case shown="True" w223 {
      tunnel: w189 -> [w322 w333]
      tunnel: w221 -> [w325 _]
      tunnel: [w321 w333] -> w169
      frame False {
        n145 = Equal To 0?(x=w322) -> (x = 0?=w326:bool)
        n146 = And(x=w326, y=w325) -> (x .and. y?=w324:bool)
        n147 = case shown="True" w324 {
          frame False {
          }
          frame True {
            w329 = FALSE ("Ack hard alarm!")
            n148 = property on="System Alarm" class="Bool (strict)"("Value"=w329) -> ()  [unwired: 2 in, 2 out]
            n149 = property on="Hard Alarm" class="Bool (strict)"("Value"=w329) -> ()  [unwired: 2 in, 2 out]
          }
        }
        n150 = case shown="False" "Acknowledge" {
          tunnel: [w327 0.0 ("Numeric")] -> w321
          tunnel: w322 -> [w327 _]
          frame False {
          }
          frame True {
          }
        }
      }
      frame True {
        n151 = local read "Table"() -> (w336:string[][])
        n152 = call "Error list.vi"("Error code"=w333, "Error array in"=w336) -> ("Hard alarm?"=w330:bool, "Error array out"=w335:string[][])  [unwired: 8 in]
        "Hard Alarm" <- w330
        "System Alarm" <- w330
        n153 = Not(x=w330) -> (.not. x?=w331:bool)
        "Soft Alarm" <- w331
        n154 = case shown="True" w331 {
          frame False {
          }
          frame True {
            n155 = property on="Alarm ack" class="Bool"("DisabledEnum"=T13."Enabled" ("Disabled")) -> ()  [unwired: 2 in, 2 out]
          }
        }
        n156 = local write "Table"(w335) -> ()
        n157 = local write "Acknowledge"(FALSE ("Acknowledge")) -> ()
        n158 = property on="Tab Control" class="TabCtl (strict)"("Value"=6) -> ()  [unwired: 2 in, 2 out]
      }
    }
    n159 = Index Array(array=w96, index #1=0 ("index"), index #2=1 ("index"), index #3=2 ("index"), index #4=3 ("index"), index #5=4 ("index"), index #6=5 ("index"), index #7=7 ("index"), index #8=8 ("index"), index #9=9 ("index"), index #10=10 ("index"), index #11=12 ("index"), index #12=13 ("index"), index #13=14 ("index"), index #14=15 ("index"), index #15=16 ("index"), index #16=17 ("index"), index #17=32 ("index"), index #18=33 ("index"), index #19=34 ("index"), index #20=35 ("index"), index #21=36 ("index"), index #22=38 ("index"), index #23=39 ("index"), index #24=40 ("index"), index #25=41 ("index"), index #26=42 ("index"), index #27=43 ("index"), index #28=44 ("index"), index #29=45 ("index"), index #30=46 ("index"), index #31=47 ("index")) -> (element #1=w154:dbl, element #2=w153:dbl, element #3=w150:dbl, element #4=w148:dbl, element #5=w149:dbl, element #6=w147:dbl, element #7=w146:dbl, element #8=w145:dbl, element #9=w144:dbl, element #10=w143:dbl, element #11=w138:dbl, element #12=w137:dbl, element #13=w136:dbl, element #14=w135:dbl, element #15=w134:dbl, element #16=w133:dbl, element #17=w127:dbl, element #18=w126:dbl, element #19=w125:dbl, element #20=w124:dbl, element #21=w123:dbl, element #22=w118:dbl, element #23=w117:dbl, element #24=w116:dbl, element #25=w115:dbl, element #26=→"Furnace temp 1":dbl, element #27=→"O2 Rapidox":dbl, element #28=w108:dbl, element #29=w107:dbl, element #30=w104:dbl, element #31=w103:dbl)
    n160 = Build Array(w157, w156) -> (w158:bool[])
    n161 = Boolean Array To Number(Boolean array=w158) -> (number=w155:u32)
    n162 = case shown="0, Default" w155 {
      tunnel: w154 -> [w279 w281 _ _]
      tunnel: w153 -> [_ w280 _ _]
      tunnel: [w279 w281 w282 w283] -> w152
      tunnel: [0.0 ("y") w280 w282 w283] -> w151
      frame 0, Default {
      }
      frame 1 {
      }
      frame 2 {
        w282 = 0.0 ("y")
      }
      frame 3 {
        w283 = 0.0 ("y")
      }
    }
    n163 = Merge Signals(w138, w137, w136, w135, w134, w133) -> (→"Sample Temperatures (°C)":dynamicdata)
    n164 = Merge Signals(w127, w126, w125, w124, w123) -> (→"System Temperatures (°C)":dynamicdata)
    n165 = Merge Signals(w108, w104) -> (→"NO Concentration (ppm)":dynamicdata)
    n166 = Merge Signals(w107, w103, w97) -> (→"Lambda":dynamicdata)
    n167 = Merge Signals(w118, w117, w116, w115) -> (→"Heat Exchanger Temperatures (°C)":dynamicdata)
    n168 = Merge Signals(w152, w151) -> (→"Flow Rate (g/s)":dynamicdata)
    n169 = Merge Signals(w150, w148, w147, w146, w145, w143) -> (→"M584L Upstream & Downstream":dynamicdata)
    n170 = Merge Signals(w149, w144) -> (→"HC Concentration (ppm)":dynamicdata)
    n171 = local read "stop 2"() -> (w216:bool)
    n172 = node-c288() -> ()  [unwired: 1 in, 1 out]
  }
  n173 = while {
    tunnel: w35 -> [w407]
    tunnel: w19 -> [w405]
    tunnel: w21 -> [w404]
    tunnel: [FALSE ("stop 2")] -> w9
    stop <- w408 stop-if-true
    n174 = Dequeue Element(queue=w407) -> (element=w406:T10)  [unwired: 2 in, 3 out]
    n175 = case shown="\"load test array\"" w406 {
      tunnel: w405 -> [_ _ _ w455 w466 w502 w536 _ _ _ _ _ _ _ w899 _ _ _ _ _ _ _]
      tunnel: w404 -> [_ _ _ _ _ _ _ _ w549 w564 w619 w664 _ _ _ _ _ _ _ _ _ _]
      frame "main", Default {
        # "0 Stop Cmd\n1 Test Number\n2 Flow Rate\n3 Start Temperature \n4 Stop Temperature\n5 Furnace Ramp Rate\n6 Inlet Lambda\n7 Inlet O2\n8 Inlet Lambda Rich\n9 Inlet Lambda Lean\n10 Inlet Temperature\n11 NO ppm SW\n12 NO ppm LO\n13 NO:CO Ratio\n14 Temperature Limit\n15 Connected???\n16 Inlet Temp Age\n17 Flow Rate Age\n18 NOx Conc\n19 CO conc %\n20 HC conc %\n21 Bleed H2O \n22 Bleed CO2\n23 Bleed N2 \n24 lambda P\n25 lambda I\n26 lambda D\n27 purge duration\n28 Target furnace lambda\n29 HC reaction ct\n30 Full system"
        # "30"
        # "25"
        # "20"
        # "15"
        # "10"
        # "5"
        # "0"
        # "15"
        # "10"
        # "5"
        # "0"
        # "Main page, pulls together information from 'Performance Set-up' page to 'Control Variables' shared variable linking to the Real-time."
        # "0 NOx Conc\n1 CO conc %\n2 HC conc %\n3 Bleed H2O \n4 Bleed CO2\n5 Bleed N2 \n6 lambda P\n7 lambda I\n8 lambda D\n9 purge duration\n10 Target furnace lambda\n11 HC reaction ct\n12 Full system\n13 Log interval\n14 MKS 1\n15 MKS 2"
        n176 = local read "output cluster"() -> (w411:T2)
        n177 = Unbundle(w411) -> ("NOx Concentration (ppm)"=w416:T1, "CO concentration %"=w415:T1, "HC concentration %"=w414:T1, "Bleed H2O %"=w413:T1, "Bleed CO2 %"=w412:T1, "Bleed N2 %"=w427:T1, "lambda P"=w426:T1, "lambda I"=w425:T1, "lambda D"=w428:T1, "Purge duration (seconds)"=w429:T1, "Target furnace lambda"=w421:T1, "HC reaction constant"=w420:T1, w422:i16, "Log interval (HRS)"=→"Log interval (seconds)":T1, →"MKS 1":i16, →"MKS 2":i16)
        n178 = local read "Test Flow Rate(g/s)"() -> (w441:T1)
        n179 = local read "Test number"() -> (w446:u16)
        n180 = local read "Connected?"() -> (w435:bool)
        n181 = local read "NO ppm Loff"() -> (w431:T1)
        n182 = local read "NO:CO Ratio"() -> (w430:T1)
        n183 = local read "Inlet LAMBDA"() -> (w433:T1)
        n184 = local read "Inlet O2 (%)"() -> (w432:T1)
        n185 = Boolean To (0,1)(Boolean=w435) -> (0, 1=w419:i16)
        n186 = Not Equal To 0?(x=w422) -> (x != 0?=→"Full system?":bool)
        n187 = Build Array("Stop Cmd", w446, w441, "Test Start Temperature (°C)", "Test Stop temperature (°C)", "Furnace Ramp Rate (°C/min)", w433, w432, "Inlet LAMBDA Rich", "Inlet LAMBDA Lean", "Inlet Temperature (°C)", "NO ppm SW", w431, w430, "Temperature Limit (°C)", w419, "Inlet temp Age", "Flow rate Age", w416, w415, w414, w413, w412, w427, w426, w425, w428, w429, w421, w420, w422) -> (w437:T1[])
        n188 = shared-variable "NI-cRIO9074-018C1D8D\\Library 1.lvlib\\Control Variables"(w437) -> ()  [unwired: 1 in, 1 out]
      }
      frame "start test" {
        w447 = FALSE
        n189 = property on="Pass" class="Bool (strict)"("Value"=w447) -> ()  [unwired: 2 in, 2 out]
        n190 = property on="Fail" class="Bool (strict)"("Value"=w447) -> ()  [unwired: 2 in, 2 out]
        n191 = local write "Pass"(w447) -> ()
        n192 = local write "Fail"(w447) -> ()
        n193 = shared-variable "NI-cRIO9074-018C1D8D\\Library 1.lvlib\\Enum 1"("Enum 1") -> ()  [unwired: 1 in, 1 out]
      }
      frame "clear table 1" {
        n194 = property on="Sub-Cycle Name" class="Str (strict)"("Value"="" ("Subcycle name")) -> ()  [unwired: 2 in, 2 out]
        n195 = local write "Flag1"(FALSE) -> ()
        n196 = local write "Sub-Cycle Pattern"(string[][] [["", "0", "", "", "", "", "", "", "", "", "", "", ""], ["", "", "", "", "", "", "", "", "", "", "", "", ""], ["", "", "", "", "", "", "", "", "", "", "", "", ""], ["", "", "", "", "", "", "", "", "", "", "", "", ""], ["", "", "", "", "", "", "", "", "", "", "", "", ""], ["", "", "", "", "", "", "", "", "", "", "", "", ""], ["", "", "", "", "", "", "", "", "", "", "", "", ""], ["", "", "", "", "", "", "", "", "", "", "", "", ""], ["", "", "", "", "", "", "", "", "", "", "", "", ""], ["", "", "", "", "", "", "", "", "", "", "", "", ""], ["", "", "", "", "", "", "", "", "", "", "", "", ""], ["", "", "", "", "", "", "", "", "", "", "", "", ""], ["", "", "", "", "", "", "", "", "", "", "", "", ""], ["", "", "", "", "", "", "", "", "", "", "", "", ""], ["", "", "", "", "", "", "", "", "", "", "", "", ""], ["", "", "", "", "", "", "", "", "", "", "", "", ""], ["", "", "", "", "", "", "", "", "", "", "", "", ""], ["", "", "", "", "", "", "", "", "", "", "", "", ""], ["", "", "", "", "", "", "", "", "", "", "", "", ""], ["", "", "", "", "", "", "", "", "", "", "", "", ""], ["", "", "", "", "", "", "", "", "", "", "", "", ""], ["", "", "", "", "", "", "", "", "", "", "", "", ""], ["", "", "", "", "", "", "", "", "", "", "", "", ""], ["", "", "", "", "", "", "", "", "", "", "", "", ""], ["", "", "", "", "", "", "", "", "", "", "", "", ""], ["", "", "", "", "", "", "", "", "", "", "", "", ""], ["", "", "", "", "", "", "", "", "", "", "", "", ""], ["", "", "", "", "", "", "", "", "", "", "", "", ""], ["", "", "", "", "", "", "", "", "", "", "", "", ""], ["", "", "", "", "", "", "", "", "", "", "", "", ""], ["", "", "", "", "", "", "", "", "", "", "", "", ""]]) -> ()
      }
      frame "update list 1" {
        n197 = String To Path(string=w455) -> (path=w454:path)
        n198 = List Folder(path=w454, pattern="*.eyes") -> (filenames=w453:string[])  [unwired: 2 in, 3 out]
        n199 = property on="Sub-Cycle List" class="LstBox (strict)"("Item Names"=w453) -> ()  [unwired: 2 in, 2 out]
      }
      frame "save subc" {
        w459 = ".eyes" ("string")
        # "Save sub-cycle routine, for ageing cycle."
        n200 = local read "Sub-Cycle Name"() -> (w458:T5)
        n201 = String To Path(string=w466) -> (path=w471:path)
        n202 = Equal?(x=w458, y="") -> (x = y?=w463:bool)
        n203 = List Folder(path=w471, pattern="*.eyes" ("string")) -> (filenames=w470:string[])  [unwired: 2 in, 3 out]
        n204 = Concatenate Strings(w458, w459) -> (w457:string)
        n205 = Concatenate Strings(w466, w458, w459) -> (w472:string)
        n206 = Search 1D Array(1D array=w470, element=w457) -> (index of element=w469:i32)  [unwired: 1 in]
        n207 = case shown="True" w463 {
          tunnel: [TRUE FALSE] -> w462
          frame False {
          }
          frame True {
            n208 = One Button Dialog(message="Insert file name!") -> ()  [unwired: 1 in, 1 out]
          }
        }
        n209 = String To Path(string=w472) -> (path=w465:path)
        n210 = Equal?(x=w469, y=-1) -> (x = y?=w467:bool)
        n211 = case shown="False" w467 {
          selector: w467 -> [_ w478]
          tunnel: [w476 w478] -> w461
          frame False {
            n212 = Two Button Dialog(message="A file with this name already exists!\nDo you want to overwrite?") -> (T button?=w476:bool)  [unwired: 2 in]
          }
          frame True {
          }
        }
        n213 = And(x=w461, y=w462) -> (x .and. y?=w460:bool)
        n214 = case shown="True" w460 {
          tunnel: w465 -> [_ w483]
          frame False {
          }
          frame True {
            n215 = local read "Sub-Cycle Pattern"() -> (w482:string[][])
            n216 = call "Table check.vi"("Input table"=w482) -> ("Incomplete?"=w480:bool, "Length"=w481:i32)  [unwired: 9 in]
            n217 = case shown="False" w480 {
              tunnel: w482 -> [w491 _]
              tunnel: w483 -> [w490 _]
              tunnel: w481 -> [w489 _]
              tunnel: string[] [] -> [w488 _]
              frame False {
                n218 = for {
                  N: w489 -> [_]
                  tunnel: w491 -> [w498]
                  shift-right: [w495] -> w487
                  shift-left: w488 -> [w496]
                  i -> [w497]
                  n219 = Index Array(array=w498, index (row)=w497) -> (element=w494:string[])  [unwired: 1 in]
                  n220 = Delete From Array(array=w494, index=0) -> (array with subset deleted=w493:string[])  [unwired: 1 in, 1 out]
                  n221 = Build Array (concatenate)(w496, w493) -> (w495:string[])
                }
                n222 = Build Array (concatenate)("SubCycle Data File for EYECAT - do not modify", w487) -> (w485:string[])
                n223 = call-poly <vilib>:"Write To Spreadsheet File.vi"("1D data"=w485, "file path (dialog if empty)"=w490) -> ()  [unwired: 6 in, 1 out]
              }
              frame True {
                n224 = One Button Dialog(message="The table is incomplete!\nplease review and save again!") -> ()  [unwired: 1 in, 1 out]
              }
            }
            n225 = local write "Flag1"(FALSE) -> ()
          }
        }
      }
      frame "load subc" {
        # "Load sub-cycle routine from table for ageing test."
        n226 = local read "Flag1"() -> (w503:bool)
        n227 = case shown="True" w503 {
          tunnel: [w530 w532] -> w501
          tunnel: w502 -> [w530 w532]
          tunnel: [TRUE w531] -> w500
          frame False {
          }
          frame True {
            n228 = Two Button Dialog(message="The table has been modified.\nDo you want to continue?") -> (T button?=w531:bool)  [unwired: 2 in]
          }
        }
        n229 = case shown="True" w500 {
          tunnel: w501 -> [_ w507]
          frame False {
          }
          frame True {
            n230 = property on="Sub-Cycle List" class="LstBox (strict)"() -> ("Item Names"=w519:string[])  [unwired: 2 in, 2 out]
            n231 = Index Array(array=w519, index="Sub-Cycle List") -> (element=w506:string)
            n232 = Concatenate Strings(w507, w506) -> (w517:string)
            n233 = Search/Split String(string=w506, search string/char (-)=".") -> (substring before match=w504:string)  [unwired: 1 in, 2 out]
            n234 = local write "Sub-Cycle Name"(w504) -> ()
            n235 = String To Path(string=w517) -> (path=w516:path)
            n236 = call-poly <vilib>:"Read From Spreadsheet File.vi"("file path (dialog if empty)"=w516) -> ("first row"=w512:string[])  [unwired: 6 in, 4 out]
            n237 = Delete From Array(array=w512, length=1, index=0) -> (array with subset deleted=w509:string[])  [unwired: 1 out]
            n238 = Array Size(array=w509) -> (size(s)=w515:i32)
            n239 = Divide(x=w515, y=12) -> (x/y=w508:dbl)
            n240 = for {
              N: w508 -> [_]
              shift-right: [w525] -> _
              shift-left: w509 -> [w528]
              tunnel: [w524] -> w513 mode=indexing
              i -> [w523]
              n241 = Increment(x=w523) -> (x+1=w522:i32)
              n242 = Delete From Array(array=w528, length=12, index=0) -> (deleted portion=w520:string[], array with subset deleted=w525:string[])
              n243 = Number To Decimal String(number=w522) -> (decimal integer string=w521:string)  [unwired: 1 in]
              n244 = Build Array (concatenate)(w521, w520) -> (w524:string[])
            }
            n245 = local write "Sub-Cycle Pattern"(w513) -> ()
          }
        }
      }
      frame "delete subc" {
        # "Delete sub-cycle from sub-cycle table for ageing test"
        n246 = Two Button Dialog(message="This operation will permanently delete this file!\nDo you want to continue?") -> (T button?=w535:bool)  [unwired: 2 in]
        n247 = case shown="True" w535 {
          tunnel: w536 -> [_ w541]
          frame False {
          }
          frame True {
            n248 = local read "Sub-Cycle List"() -> (w538:i32)
            n249 = property on="Sub-Cycle List" class="LstBox (strict)"() -> ("Item Names"=w539:string[])  [unwired: 2 in, 2 out]
            n250 = Index Array(array=w539, index=w538) -> (element=w543:string)
            n251 = Concatenate Strings(w541, w543) -> (w542:string)
            n252 = local write "Flag1"(FALSE) -> ()
            n253 = String To Path(string=w542) -> (path=w540:path)
            n254 = Delete(path (use dialog)=w540) -> ()  [unwired: 4 in, 3 out]
          }
        }
      }
      frame "clear table 2" {
        n255 = property on="Cycle Name" class="Str (strict)"("Value"="" ("Subcycle name")) -> ()  [unwired: 2 in, 2 out]
        n256 = local write "Flag 2"(FALSE) -> ()
        n257 = local write "Cycle Pattern"(string[][] [["", "", "", "", ""], ["", "", "", "", ""], ["", "", "", "", ""], ["", "", "", "", ""], ["", "", "", "", ""], ["", "", "", "", ""], ["", "", "", "", ""], ["", "", "", "", ""], ["", "", "", "", ""], ["", "", "", "", ""], ["", "", "", "", ""], ["", "", "", "", ""], ["", "", "", "", ""], ["", "", "", "", ""], ["", "", "", "", ""], ["", "", "", "", ""], ["", "", "", "", ""], ["", "", "", "", ""], ["", "", "", "", ""], ["", "", "", "", ""], ["", "", "", "", ""], ["", "", "", "", ""], ["", "", "", "", ""], ["", "", "", "", ""], ["", "", "", "", ""], ["", "", "", "", ""], ["", "", "", "", ""], ["", "", "", "", ""], ["", "", "", "", ""], ["", "", "", "", ""], ["", "", "", "", ""]]) -> ()
      }
      frame "update list 2" {
        n258 = String To Path(string=w549) -> (path=w550:path)
        n259 = List Folder(path=w550, pattern="*.eyec") -> (filenames=w548:string[])  [unwired: 2 in, 3 out]
        n260 = property on="Cycle List" class="LstBox (strict)"("Item Names"=w548) -> ()  [unwired: 2 in, 2 out]
      }
      frame "save cycle" {
        w551 = ".eyec" ("string")
        n261 = local read "Cycle Name"() -> (w552:T5)
        n262 = String To Path(string=w564) -> (path=w565:path)
        n263 = List Folder(path=w565, pattern="*.eyec" ("string")) -> (filenames=w563:string[])  [unwired: 2 in, 3 out]
        n264 = Equal?(x=w552, y="") -> (x = y?=w558:bool)
        n265 = Concatenate Strings(w552, w551) -> (w554:string)
        n266 = Search 1D Array(1D array=w563, element=w554) -> (index of element=w562:i32)  [unwired: 1 in]
        n267 = Concatenate Strings(w564, w552, w551) -> (w567:string)
        n268 = case shown="True" w558 {
          tunnel: [TRUE FALSE] -> w556
          frame False {
          }
          frame True {
            n269 = One Button Dialog(message="Insert file name!") -> ()  [unwired: 1 in, 1 out]
          }
        }
        n270 = String To Path(string=w567) -> (path=w566:path)
        n271 = Equal?(x=w562, y=-1) -> (x = y?=w560:bool)
        n272 = case shown="False" w560 {
          selector: w560 -> [_ w616]
          tunnel: [w614 w616] -> w557
          frame False {
            n273 = Two Button Dialog(message="A file with this name already exists!\nDo you want to overwrite?") -> (T button?=w614:bool)  [unwired: 2 in]
          }
          frame True {
          }
        }
        n274 = And(x=w557, y=w556) -> (x .and. y?=w555:bool)
        n275 = case shown="True" w555 {
          tunnel: w566 -> [_ w574]
          frame False {
          }
          frame True {
            n276 = local read "Cycle Pattern"() -> (w573:string[][])
            n277 = call "Table check.vi"("Input table"=w573) -> ("Incomplete?"=w571:bool, "Length"=w572:i32)  [unwired: 9 in]
            n278 = case shown="False" w571 {
              tunnel: w574 -> [w583 _]
              tunnel: w573 -> [w582 _]
              tunnel: w572 -> [w575 _]
              frame False {
                n279 = Number To Decimal String(number=w575) -> (decimal integer string=w578:string)  [unwired: 1 in]
                n280 = for {
                  N: w575 -> [_]
                  tunnel: w582 -> [w612]
                  shift-right: [w600] -> w579
                  shift-left: string[] [] -> [w610]
                  i -> [w611]
                  w591 = 12 ("length")
                  n281 = Index Array(array=w612, index (row)=w611) -> (element=w606:string[])  [unwired: 1 in]
                  n282 = Index Array(array=w606, index=3) -> (element=w596:string)
                  n283 = Index Array(array=w606, index=1) -> (element=w595:string)
                  n284 = Concatenate Strings("C:\\Setup Files\\Subcycles Folder\\", w595) -> (w607:string)
                  n285 = String To Path(string=w607) -> (path=w608:path)
                  n286 = call-poly <vilib>:"Read From Spreadsheet File.vi"("file path (dialog if empty)"=w608) -> ("first row"=w599:string[])  [unwired: 6 in, 4 out]
                  n287 = Delete From Array(array=w599, length=1, index=0) -> (array with subset deleted=w593:string[])  [unwired: 1 out]
                  n288 = String Length(string=w593) -> (length=w602:i32[])
                  n289 = Array Size(array=w602) -> (size(s)=w594:i32)
                  n290 = Divide(x=w594, y=w591) -> (x/y=w592:dbl)
                  n291 = Decrement(x=w592) -> (x-1=w584:dbl)
                  n292 = Multiply(x=w591, y=w584) -> (x*y=w590:dbl)
                  n293 = Number To Decimal String(number=w584) -> (decimal integer string=w601:string)  [unwired: 1 in]
                  n294 = Delete From Array(array=w593, length=12, index=w590) -> (deleted portion=w587:string[], array with subset deleted=w588:string[])
                  n295 = Index Array(array=w587, index=0) -> (element=w585:string)
                  n296 = Build Array (concatenate)(w595, w596, w601, w585, w588) -> (w605:string[])
                  n297 = Build Array (concatenate)(w610, w605) -> (w600:string[])
                }
                n298 = local write "Flag 2"(FALSE) -> ()
                n299 = Build Array (concatenate)("Cycle Data File for EYECAT - do not modify", w578, w579) -> (w580:string[])
                n300 = call-poly <vilib>:"Write To Spreadsheet File.vi"("1D data"=w580, "file path (dialog if empty)"=w583) -> ()  [unwired: 6 in, 1 out]
              }
              frame True {
                n301 = One Button Dialog(message="The table is incomplete!\nplease review and save again!") -> ()  [unwired: 1 in, 1 out]
              }
            }
          }
        }
      }
      frame "load cycle" {
        # "Load ageing 'cycle' for ageing routine."
        n302 = local read "Flag 2"() -> (w620:bool)
        n303 = case shown="True" w620 {
          tunnel: [w659 w661] -> w617
          tunnel: w619 -> [w659 w661]
          tunnel: [TRUE ("T button?") w660] -> w618
          frame False {
          }
          frame True {
            n304 = Two Button Dialog(message="The table has been modified.\nDo you want to continue?") -> (T button?=w660:bool)  [unwired: 2 in]
          }
        }
        n305 = case shown="True" w618 {
          tunnel: w617 -> [_ w623]
          frame False {
          }
          frame True {
            n306 = property on="Cycle List" class="LstBox (strict)"() -> ("Item Names"=w639:string[])  [unwired: 2 in, 2 out]
            n307 = Index Array(array=w639, index="Cycle List") -> (element=w625:string)
            n308 = Concatenate Strings(w623, w625) -> (w638:string)
            n309 = Search/Split String(string=w625, search string/char (-)=".") -> (substring before match=w624:string)  [unwired: 1 in, 2 out]
            n310 = String To Path(string=w638) -> (path=w637:path)
            n311 = local write "Cycle Name"(w624) -> ()
            n312 = call-poly <vilib>:"Read From Spreadsheet File.vi"("file path (dialog if empty)"=w637) -> ("first row"=w621:string[])  [unwired: 6 in, 4 out]
            n313 = Delete From Array(array=w621, length=2, index=0) -> (array with subset deleted=w622:string[])  [unwired: 1 out]
            n314 = Index Array(array=w621, index=1) -> (element=w636:string)
            n315 = Decimal String To Number(string=w636) -> (number=w635:i32)  [unwired: 2 in, 1 out]
            n316 = for {
              N: w635 -> [_]
              tunnel: w622 -> [w657]
              tunnel: [w652] -> w630 mode=indexing
              shift-right: [w642] -> _
              shift-left: 0 ("x") -> [w643]
              i -> [w656]
              w653 = ""
              n317 = Increment(x=w643) -> (x+1=w641:i32)
              n318 = Increment(x=w641) -> (x+1=w649:i32)
              n319 = Increment(x=w656) -> (x+1=w651:i32)
              n320 = Number To Decimal String(number=w651) -> (decimal integer string=w650:string)  [unwired: 1 in]
              n321 = Index Array(array=w657, index #1=w643, index #2=w641, index #3=w649) -> (element #1=w655:string, element #2=w654:string, element #3=w648:string)
              n322 = Build Array(w650, w655, w653, w654, w653) -> (w652:string[])
              n323 = Decimal String To Number(string=w648) -> (number=w647:i32)  [unwired: 2 in, 1 out]
              n324 = Multiply(x=w647, y=12 ("x")) -> (x*y=w645:i32)
              n325 = Compound Arithmetic op=ADD(w645, 4, w643) -> (w642:i32)
            }
            n326 = Insert Into Array(array=string[][] [["", "", "", "", ""], ["", "", "", "", ""], ["", "", "", "", ""], ["", "", "", "", ""], ["", "", "", "", ""], ["", "", "", "", ""], ["", "", "", "", ""], ["", "", "", "", ""], ["", "", "", "", ""], ["", "", "", "", ""], ["", "", "", "", ""], ["", "", "", "", ""], ["", "", "", "", ""], ["", "", "", "", ""], ["", "", "", "", ""], ["", "", "", "", ""], ["", "", "", "", ""], ["", "", "", "", ""], ["", "", "", "", ""], ["", "", "", "", ""], ["", "", "", "", ""], ["", "", "", "", ""], ["", "", "", "", ""], ["", "", "", "", ""], ["", "", "", "", ""], ["", "", "", "", ""], ["", "", "", "", ""], ["", "", "", "", ""], ["", "", "", "", ""], ["", "", "", "", ""], ["", "", "", "", ""]], index (row)=0, new element=w630) -> (w629:string[][])  [unwired: 1 in]
            n327 = local write "Cycle Pattern"(w629) -> ()
          }
        }
      }
      frame "delete cycle" {
        # "Delete ageing test cycle from table, ageing test tab"
        n328 = Two Button Dialog(message="This operation will permanently delete this file!\nDo you want to continue?") -> (T button?=w665:bool)  [unwired: 2 in]
        n329 = case shown="True" w665 {
          tunnel: w664 -> [_ w670]
          frame False {
          }
          frame True {
            n330 = local read "Cycle List"() -> (w671:i32)
            n331 = property on="Cycle List" class="LstBox (strict)"() -> ("Item Names"=w672:string[])  [unwired: 2 in, 2 out]
            n332 = Index Array(array=w672, index=w671) -> (element=w669:string)
            n333 = Concatenate Strings(w670, w669) -> (w668:string)
            n334 = String To Path(string=w668) -> (path=w667:path)
            n335 = Delete(path (use dialog)=w667) -> ()  [unwired: 4 in, 3 out]
            n336 = local write "Flag 2"(FALSE) -> ()
          }
        }
      }
      frame "calc HC CO" {
        # "Calculates HC and CO in ageing test sub-cyclce, for ageing test. (ageing test tab)"
        n337 = local read "Sub-Cycle Pattern"() -> (w689:string[][])
        n338 = Index Array(array=w689, index (col) #1=3 ("disabled index (col)"), index (col) #2=4 ("index (col)"), index (col) #3=11 ("index (col)")) -> (element #1=w679:string[], element #2=w686:string[], element #3=w673:string[])  [unwired: 3 in]
        n339 = Array Size(array=w679) -> (size(s)=w677:i32)
        n340 = Search 1D Array(1D array=w679, element="") -> (index of element=w676:i32)  [unwired: 1 in]
        n341 = Equal?(x=w676, y=-1) -> (x = y?=w678:bool)
        n342 = Select(t=w677, s=w678, f=w676) -> (s? t:f=w675:i32)
        n343 = for {
          N: w675 -> [_]
          tunnel: [w700] -> w683 mode=indexing
          tunnel: [w699] -> w682 mode=indexing
          tunnel: w679 -> [w698] mode=indexing
          tunnel: w686 -> [w697] mode=indexing
          tunnel: w673 -> [w696] mode=indexing
          w695 = ""
          n344 = Not Equal?(x=w698, y=w695) -> (x != y?=w694:bool)
          n345 = Not Equal?(x=w697, y=w695) -> (x != y?=w693:bool)
          n346 = Not Equal?(x=w696, y=w695) -> (x != y?=w692:bool)
          n347 = Compound Arithmetic op=AND(w694, w693, w692) -> (w691:bool)
          n348 = case shown="True" w691 {
            tunnel: w698 -> [_ w729]
            tunnel: w697 -> [_ w728]
            tunnel: [w701 w725] -> w699
            tunnel: [w701 w724] -> w700
            tunnel: w696 -> [_ w702]
            frame False {
              w701 = ""
            }
            frame True {
              # "O2Eq"
              n349 = Fract/Exp String To Number(string=w702) -> (number=w703:dbl)  [unwired: 3 in, 1 out]
              n350 = Fract/Exp String To Number(string=w729) -> (number=w710:dbl)  [unwired: 3 in, 1 out]
              n351 = Fract/Exp String To Number(string=w728) -> (number=w706:dbl)  [unwired: 3 in, 1 out]
              n352 = Decrement(x=w710) -> (x-1=w711:dbl)
              n353 = Divide(x=w703, y=20000.0) -> (x/y=w704:dbl)
              n354 = Multiply(x=4.76, y=w710) -> (x*y=w715:dbl)
              n355 = Multiply(x=w711, y=100.0) -> (x*y=w713:dbl)
              n356 = Add(x=w706, y=w704) -> (x+y=w707:dbl)
              n357 = Add(x=0.33, y=w715) -> (x+y=w717:dbl)
              n358 = Divide(x=w713, y=w717) -> (x/y=w718:dbl)
              n359 = Subtract(x=w707, y=w718) -> (x-y=w720:dbl)
              n360 = Multiply(x=w720, y=2.0) -> (x*y=w708:dbl)
              n361 = Divide(x=w720, y=5.0) -> (x/y=w709:dbl)
              n362 = Number To Fractional String(number=w709, width (-)=i16 6, precision (6)=i16 3) -> (F-format string=w724:string)  [unwired: 1 in]
              n363 = Number To Fractional String(number=w708, width (-)=i16 6, precision (6)=i16 2) -> (F-format string=w725:string)  [unwired: 1 in]
            }
          }
        }
        n364 = Replace Array Subset(array=w689, new element #1=w683, index (col) #1=5 ("disabled index (col)"), new element #2=w682, index (col) #2=6 ("disabled index (col)")) -> (w687:string[][])  [unwired: 2 in]
        n365 = local write "Sub-Cycle Pattern"(w687) -> ()
      }
      frame "Total time calc" {
        w744 = i16 2 ("width (-)")
        w751 = ":"
        # "Calculates the total time required for the test based on the length of sub-cycle and number of repeats."
        n366 = local read "Cycle Pattern"() -> (w758:string[][])
        n367 = Index Array(array=w758, index (col)=4 ("disabled index (col)")) -> (element=w731:string[])  [unwired: 1 in]
        n368 = Array Size(array=w731) -> (size(s)=w733:i32)
        n369 = Search 1D Array(1D array=w731, element="") -> (index of element=w732:i32)  [unwired: 1 in]
        n370 = Equal?(x=w732, y=-1) -> (x = y?=w734:bool)
        n371 = Select(t=w733, s=w734, f=w732) -> (s? t:f=w730:i32)
        n372 = for {
          N: w730 -> [_]
          tunnel: w731 -> [w766] mode=indexing
          shift-right: [w768] -> w754
          shift-left: 0 -> [w769]
          n373 = xnode "Match Regular Expression"("input string"=w766, "regular expression"=":" ("search string/char (-)")) -> ("before match"=w765:string, "after match"=w762:string)  [unwired: 4 in, 3 out]
          n374 = Decimal String To Number(string=w765) -> (number=w764:i32)  [unwired: 2 in, 1 out]
          n375 = Decimal String To Number(string=w762) -> (number=w761:i32)  [unwired: 2 in, 1 out]
          n376 = Multiply(x=w764, y=60) -> (x*y=w760:i32)
          n377 = Add(x=w760, y=w761) -> (x+y=w759:i32)
          n378 = Add(x=w759, y=w769) -> (x+y=w768:i32)
        }
        n379 = local read "Total Number of Cycles"() -> (w755:T1)
        n380 = Multiply(x=w754, y=w755) -> (x*y=w750:T1)
        n381 = Quotient & Remainder(x=w750, y=3600.0) -> (x-y*floor(x/y)=w737:T1, floor(x/y)=w747:T1)
        n382 = Quotient & Remainder(x=w737, y=60.0) -> (x-y*floor(x/y)=w745:T1, floor(x/y)=w746:T1)
        n383 = Number To Decimal String(number=w747) -> (decimal integer string=w752:string)  [unwired: 1 in]
        n384 = Number To Decimal String(number=w746, width (-)=w744) -> (decimal integer string=w748:string)
        n385 = Number To Decimal String(number=w745, width (-)=w744) -> (decimal integer string=w743:string)
        n386 = Concatenate Strings(w752, w751, w748, w751, w743) -> (w742:string)
        n387 = call <vilib>:"Search and Replace Pattern.vi"("string"=w742, "regular expression (\"\")"=" " ("replace string (\"\")"), "replace string (\"\")"="0" ("replace string (\"\")"), "replace all? (F)"=TRUE) -> ("result string"=→"Total Test Duration (hrs)":string)  [unwired: 1 in, 1 out]
      }
      frame "update Cycle pattern " {
        n388 = local read "Cycle Pattern"() -> (w897:string[][])
        n389 = Index Array(array=w897, index (col)=1 ("disabled index (col)")) -> (element=w882:string[])  [unwired: 1 in]
        n390 = String To Path(string=w899) -> (path=w900:path)
        n391 = Array Size(array=w882) -> (size(s)=w885:i32)
        n392 = Search 1D Array(1D array=w882, element="") -> (index of element=w884:i32)  [unwired: 1 in]
        n393 = List Folder(path=w900, pattern="*.eyes") -> (filenames=w898:string[])  [unwired: 2 in, 3 out]
        n394 = Equal?(x=w884, y=-1) -> (x = y?=w886:bool)
        n395 = Select(t=w885, s=w886, f=w884) -> (s? t:f=w883:i32)
        n396 = for {
          N: w883 -> [_]
          tunnel: w897 -> [w916] mode=indexing
          tunnel: w899 -> [w909]
          tunnel: [w911] -> w892 mode=indexing
          tunnel: [w913] -> w896 mode=indexing
          tunnel: [w910] -> w893 mode=indexing
          tunnel: w898 -> [w908]
          tunnel: [w903] -> w889 mode=indexing
          n397 = Index Array(array=w916, index #1=1 ("index"), index #2=3 ("index")) -> (element #1=w907:string, element #2=w912:string)
          n398 = Search 1D Array(1D array=w908, element=w907) -> (index of element=w906:i32)  [unwired: 1 in]
          n399 = Not Equal?(x=w906, y=-1) -> (x != y?=w904:bool)
          n400 = case shown="True" w904 {
            tunnel: [w920 w934] -> w913
            tunnel: w912 -> [_ w930]
            tunnel: [w920 w928] -> w911
            tunnel: [w920 w927] -> w910
            tunnel: w909 -> [_ w926]
            tunnel: w907 -> [w919 w925]
            tunnel: [w918 w925] -> w903
            frame False {
              w920 = "N/A" ("String")
              n401 = Concatenate Strings(w919, " - File NOT AVAILABLE !!!" ("string")) -> (w918:string)
            }
            frame True {
              w938 = i16 2 ("width (-)")
              n402 = Concatenate Strings(w926, w925) -> (w956:string)
              n403 = String To Path(string=w956) -> (path=w955:path)
              n404 = call <vilib>:"Search and Replace Pattern.vi"("string"=w930, "regular expression (\"\")"="[a-x ]" ("format string"), "replace string (\"\")"="", "replace all? (F)"=TRUE) -> ("result string"=w927:string)  [unwired: 1 in, 1 out]
              n405 = call-poly <vilib>:"Read From Spreadsheet File.vi"("file path (dialog if empty)"=w955) -> ("first row"=w924:string[])  [unwired: 6 in, 4 out]
              n406 = Delete From Array(array=w924, length=1, index=0) -> (array with subset deleted=w923:string[])  [unwired: 1 out]
              n407 = Array Size(array=w923) -> (size(s)=w954:i32)
              n408 = Equal?(x=w927, y="") -> (x = y?=w942:bool)
              n409 = Subtract(x=w954, y=12) -> (x-y=w952:i32)
              n410 = Select(t="0", s=w942, f=w927) -> (s? t:f=w941:string)
              n411 = Index Array(array=w923, index=w952) -> (element=w928:string)
              n412 = Decimal String To Number(string=w941) -> (number=w951:i32)  [unwired: 2 in, 1 out]
              n413 = Decimal String To Number(string=w928) -> (number=w950:i32)  [unwired: 2 in, 1 out]
              n414 = Multiply(x=w951, y=w950) -> (x*y=w949:i32)
              n415 = Quotient & Remainder(x=w949, y=60) -> (x-y*floor(x/y)=w947:i32, floor(x/y)=w946:i32)
              n416 = Number To Decimal String(number=w947, width (-)=w938) -> (decimal integer string=w944:string)
              n417 = Number To Decimal String(number=w946, width (-)=w938) -> (decimal integer string=w943:string)
              n418 = Concatenate Strings(w943, ":", w944) -> (w937:string)
              n419 = call <vilib>:"Search and Replace Pattern.vi"("string"=w937, "regular expression (\"\")"=" " ("replace string (\"\")"), "replace string (\"\")"="0" ("replace string (\"\")"), "replace all? (F)"=TRUE) -> ("result string"=w934:string)  [unwired: 1 in, 1 out]
            }
          }
        }
        n420 = Replace Array Subset(array=w897, new element #1=w889, index (col) #1=1 ("disabled index (col)"), new element #2=w892, index (col) #2=2 ("disabled index (col)"), new element #3=w893, index (col) #3=3 ("disabled index (col)"), new element #4=w896, index (col) #4=4 ("disabled index (col)")) -> (w901:string[][])  [unwired: 4 in]
        n421 = local write "Cycle Pattern"(w901) -> ()
      }
      frame "load cycle name" {
        n422 = property on="Cycle Pattern" class="Tbl (strict)"() -> ("EditPos"=w962:T3)  [unwired: 2 in, 2 out]
        n423 = Unbundle By Name(w962) -> ("Row"=w960:i32, "Column"=w959:i32)
        n424 = local read "Cycle Pattern"() -> (w958:string[][])
        n425 = call "SubCycles list.vi"() -> ("Subcycle name"=w961:string)  [unwired: 10 in, 1 out]
        n426 = Replace Array Subset(array=w958, new element=w961, index (row)=w960, index (col)=w959) -> (w957:string[][])
        n427 = local write "Cycle Pattern"(w957) -> ()
      }
      frame "load test array" {
        # "Loads cycle/sub-cycle from windows folder into a strings, adding ageing gas and number of cycles/time of test into an array. Array linked to shared variable 'Ageing Variables'. Passed to Real-Time inputs"
        n428 = local read "Total Test Duration (hrs)"() -> (w970:T8)
        n429 = local read "Cycle Name"() -> (w966:T5)
        n430 = Not Equal?(x=w970, y="0:00:00") -> (x != y?=w964:bool)
        n431 = Equal?(x=w966, y="") -> (x = y?=w965:bool)
        n432 = Or(x=w964, y=w965) -> (x .or. y?=w963:bool)
        n433 = case shown="True" w963 {
          selector: w963 -> [w971 _]
          tunnel: [FALSE TRUE] -> w968
          frame False {
            n434 = case shown="False" w971 {
              frame False {
                n435 = One Button Dialog(message="Incomplete Data!\nReview the cycle pattern!") -> ()  [unwired: 1 in, 1 out]
              }
              frame True {
              }
            }
          }
          frame True {
            w977 = 0.0 ("default (0 I32)")
            n436 = local read "Cycle Name"() -> (w992:T5)
            n437 = Concatenate Strings("C:\\Setup Files\\Cycles Folder\\", w992, ".eyec" ("string")) -> (w990:string)
            n438 = String To Path(string=w990) -> (path=w991:path)
            n439 = local read "Total Number of Cycles"() -> (w988:T1)
            n440 = call-poly <vilib>:"Read From Spreadsheet File.vi"("file path (dialog if empty)"=w991) -> ("first row"=w974:string[])  [unwired: 6 in, 4 out]
            n441 = call "Remove names.vi"("Array in"=w974) -> ("Array out"=w983:string[])  [unwired: 10 in]
            n442 = Index Array(array=w974, index #1=14 ("index"), index #2=15 ("index")) -> (element #1=w979:string, element #2=w975:string)
            n443 = Number To Decimal String(number="Ageing Gas") -> (decimal integer string=w987:string)  [unwired: 1 in]
            n444 = Number To Decimal String(number=w988) -> (decimal integer string=w986:string)  [unwired: 1 in]
            n445 = Decimal String To Number(string=w975, default (0L)=w977) -> (number=w976:dbl)  [unwired: 1 in, 1 out]
            n446 = Decimal String To Number(string=w979, default (0L)=w977) -> (number=w978:dbl)  [unwired: 1 in, 1 out]
            n447 = property on="Inlet temp Age" class="DigNum (strict)"("Value"=w978) -> ()  [unwired: 2 in, 2 out]
            n448 = property on="Flow rate Age" class="DigNum (strict)"("Value"=w976) -> ()  [unwired: 2 in, 2 out]
            n449 = Build Array (concatenate)(w987, w986, w983) -> (w982:string[])
            n450 = shared-variable "NI-cRIO9074-018C1D8D\\Library 1.lvlib\\Ageing Variables"(w982) -> ()  [unwired: 1 in, 1 out]
          }
        }
        "Test Compiled" <- w968
      }
      frame "convert to num" {
        # "Reads input array and removes any letters in array/string"
        n451 = local read "EditPos Subc"() -> (w997:T3)
        n452 = Unbundle By Name(w997) -> ("Row"=w998:i32, "Column"=w995:i32)
        n453 = Equal?(x=w995, y=7) -> (x = y?=w994:bool)
        n454 = case shown="False" w994 {
          tunnel: w998 -> [_ w1003]
          tunnel: w995 -> [_ w1001]
          tunnel: w997 -> [_ _]
          frame True {
          }
          frame False {
            n455 = local read "Sub-Cycle Pattern"() -> (w1000:string[][])
            n456 = call "Conv to num.vi"("Column"=w1001, "Row"=w1003, "Array"=w1000) -> ("result string"=w1002:string)  [unwired: 8 in]
            n457 = Replace Array Subset(array=w1000, new element=w1002, index (row)=w1003, index (col)=w1001) -> (w999:string[][])
            n458 = local write "Sub-Cycle Pattern"(w999) -> ()
          }
        }
      }
      frame "check scycle name" {
        # "Checks sub-cycle name allowing characters 0-9, a-z, A-Z. Removes all other characters from name."
        n459 = local read "Sub-Cycle Name"() -> (w1004:T5)
        n460 = call <vilib>:"Search and Replace Pattern.vi"("string"=w1004, "regular expression (\"\")"="[^0-9a-zA-Z ]" ("format string"), "replace string (\"\")"="", "replace all? (F)"=TRUE) -> ("result string"=w1010:string)  [unwired: 1 in, 1 out]
        n461 = Not Equal?(x=w1010, y=w1004) -> (x != y?=w1009:bool)
        n462 = case shown="True" w1009 {
          tunnel: w1010 -> [w1011 w1012]
          tunnel: [w1011 w1012] -> w1005
          frame False {
          }
          frame True {
            n463 = One Button Dialog(message="Unsuitable character for the file name!") -> ()  [unwired: 1 in, 1 out]
          }
        }
        n464 = local write "Sub-Cycle Name"(w1005) -> ()
      }
      frame "check cycle name" {
        # "Checks cycle name allowing characters 0-9, a-z, A-Z. Removes all other characters from name."
        n465 = local read "Cycle Name"() -> (w1014:T5)
        n466 = call <vilib>:"Search and Replace Pattern.vi"("string"=w1014, "regular expression (\"\")"="[^0-9a-zA-Z ]" ("format string"), "replace string (\"\")"="", "replace all? (F)"=TRUE) -> ("result string"=w1020:string)  [unwired: 1 in, 1 out]
        n467 = Not Equal?(x=w1020, y=w1014) -> (x != y?=w1019:bool)
        n468 = case shown="False" w1019 {
          tunnel: w1020 -> [w1021 w1022]
          tunnel: [w1021 w1022] -> w1015
          frame False {
          }
          frame True {
            n469 = One Button Dialog(message="Unsuitable character for the file name!") -> ()  [unwired: 1 in, 1 out]
          }
        }
        n470 = local write "Cycle Name"(w1015) -> ()
      }
      frame "Multigas connect" {
        n471 = flat-sequence {
          frame #0 {
            "Connected?" <- TRUE
          }
        }
      }
      frame "Multigas disconnect" {
      }
    }
    n472 = local read "stop 2"() -> (w408:bool)
  }
  n473 = while {
    tunnel: w35 -> [w1029]
    shift-right: [w1027] -> _
    shift-left: _ -> [w1026]
    stop <- w1025 stop-if-true
    n474 = event shown="[21] \"Start Test Button\": Value Change" {
      selector: _ -> [_ _ _ _ _ _ _ _ _ _ _ _ _ _ _ _ _ _ _ _ _ _ _ _ _ _ _ _]
      dyn-events: _ -> [_ _ _ _ _ _ _ _ _ _ _ _ _ _ _ _ _ _ _ _ _ _ _ _ _ _ _ _]
      timeout: 100 -> [_ _ _ _ _ _ _ _ _ _ _ _ _ _ _ _ _ _ _ _ _ _ _ _ _ _ _ _]
      tunnel: w1029 -> [w1032 w1034 _ w1043 w1051 w1058 w1065 w1076 w1080 w1091 w1096 w1099 w1104 w1126 w1134 w1135 _ _ _ _ w1179 w1188 w1212 w1230 _ w1244 _ _]
      tunnel: [w1030 w1033 _ w1044 w1050 w1057 w1064 w1075 w1078 w1086 w1093 w1098 w1102 w1123 _ _ _ _ _ _ _ _ _ _ _ _ _ _] -> w1027
      tunnel: w1026 -> [w1030 w1033 _ w1044 w1050 w1057 w1063 w1075 w1078 w1086 w1093 w1098 w1102 w1123 _ _ _ _ _ _ _ _ _ _ _ _ _ _]
      tunnel: [_ _ w1036 _ _ _ _ _ _ _ _ _ _ _ _ _ _ _ _ _ _ _ _ _ _ _ _ _] -> w1025
      event Timeout {
        n475 = event-data() -> ()  [unwired: 1 in, 2 out]
        n476 = Enqueue Element(queue=w1032, element=Control_3."main" ("Enum")) -> ()  [unwired: 2 in, 3 out]
      }
      event "Clear subcycle": Value Change {
        n477 = event-data() -> ()  [unwired: 1 in, 5 out]
        n478 = Enqueue Element(queue=w1034, element=Control_3."clear table 1" ("Enum")) -> ()  [unwired: 2 in, 3 out]
      }
      event Panel Close? {
        n479 = event-data() -> ()  [unwired: 1 in, 3 out]
        n480 = Two Button Dialog(message="This command will close Eyecat!\nDo you wish to continue?", 1:"No" ("F button name (\"Cancel\")"), 2:"Yes" ("T button name (\"OK\")")) -> (T button?=w1036:bool)
        n481 = Not(x=w1036) -> (.not. x?=w1037:bool)
        n482 = event-data("Discard?"=w1037) -> ()  [unwired: 1 in, 1 out]
      }
      event "Save sCycle": Value Change {
        n483 = event-data() -> ()  [unwired: 1 in, 5 out]
        n484 = local read "Sub-Cycle Pattern"() -> (w1041:string[][])
        n485 = call "Time column check.vi"("Array"=w1041) -> ("Mistake?"=w1042:bool)  [unwired: 10 in]
        n486 = case shown="True" w1042 {
          tunnel: w1043 -> [w1045 _]
          frame False {
            n487 = Enqueue Element(queue=w1045, element=Control_3."save subc") -> (queue out=w1047:refnum<queue>)  [unwired: 2 in, 2 out]
            n488 = Enqueue Element(queue=w1047, element=Control_3."update list 1") -> ()  [unwired: 2 in, 3 out]
          }
          frame True {
            n489 = One Button Dialog(message="The time sequence is incorrect!\nReview and save again!") -> ()  [unwired: 1 in, 1 out]
          }
        }
      }
      event "Load sCycle": Value Change {
        n490 = event-data() -> ()  [unwired: 1 in, 5 out]
        n491 = Enqueue Element(queue=w1051, element=Control_3."load subc") -> ()  [unwired: 2 in, 3 out]
      }
      event "Delete sCycle": Value Change {
        n492 = event-data() -> ()  [unwired: 1 in, 5 out]
        n493 = Enqueue Element(queue=w1058, element=Control_3."delete subc") -> (queue out=w1060:refnum<queue>)  [unwired: 2 in, 2 out]
        n494 = Enqueue Element(queue=w1060, element=Control_3."update list 1") -> (queue out=w1056:refnum<queue>)  [unwired: 2 in, 2 out]
        n495 = Enqueue Element(queue=w1056, element=Control_3."update Cycle pattern ") -> (queue out=w1053:refnum<queue>)  [unwired: 2 in, 2 out]
        n496 = Enqueue Element(queue=w1053, element=Control_3."Total time calc") -> ()  [unwired: 2 in, 3 out]
      }
      event "Sub-Cycle Pattern": Mouse Down; "Sub-Cycle Pattern": Value Change {
        n497 = event-data() -> ()  [unwired: 1 in, 3 out]
        n498 = property on="Sub-Cycle Pattern" class="Tbl (strict)"() -> ("EditPos"=w1064:T3)  [unwired: 2 in, 2 out]
        n499 = Unbundle By Name(w1064) -> ("Row"=w1066:i32)  [unwired: 1 out]
        n500 = Less?(x=w1066, y=30) -> (x < y?=w1068:bool)
        n501 = case shown="True" w1068 {
          tunnel: w1065 -> [_ w1073]
          frame False {
            n502 = One Button Dialog(message="This table is limited to 30 entries!") -> ()  [unwired: 1 in, 1 out]
          }
          frame True {
            n503 = Enqueue Element(queue=w1073, element=Control_3."convert to num") -> (queue out=w1072:refnum<queue>)  [unwired: 2 in, 2 out]
            n504 = Enqueue Element(queue=w1072, element=Control_3."calc HC CO") -> ()  [unwired: 2 in, 3 out]
          }
        }
        "EditPos Subc" <- w1063
        "Flag1" <- TRUE
      }
      event "Clear Cycle Pattern": Value Change {
        n505 = event-data() -> ()  [unwired: 1 in, 5 out]
        n506 = Enqueue Element(queue=w1076, element=Control_3."clear table 2" ("Enum")) -> ()  [unwired: 2 in, 3 out]
        n507 = local write "Test Compiled"(FALSE ("Test Compiled")) -> ()
      }
      event "Save Cycle": Value Change {
        n508 = event-data() -> ()  [unwired: 1 in, 5 out]
        n509 = Enqueue Element(queue=w1080, element=Control_3."update Cycle pattern ") -> (queue out=w1079:refnum<queue>)  [unwired: 2 in, 2 out]
        n510 = Enqueue Element(queue=w1079, element=Control_3."save cycle") -> (queue out=w1083:refnum<queue>)  [unwired: 2 in, 2 out]
        n511 = Enqueue Element(queue=w1083, element=Control_3."update list 2") -> ()  [unwired: 2 in, 3 out]
      }
      event "Load Cycle": Value Change {
        n512 = event-data() -> ()  [unwired: 1 in, 5 out]
        n513 = Enqueue Element(queue=w1091, element=Control_3."load cycle") -> (queue out=w1089:refnum<queue>)  [unwired: 2 in, 2 out]
        n514 = Enqueue Element(queue=w1089, element=Control_3."update Cycle pattern ") -> (queue out=w1088:refnum<queue>)  [unwired: 2 in, 2 out]
        n515 = local write "Test Compiled"(FALSE ("Test Compiled")) -> ()
        n516 = Enqueue Element(queue=w1088, element=Control_3."Total time calc") -> ()  [unwired: 2 in, 3 out]
      }
      event "Delete Cycle": Value Change {
        n517 = event-data() -> ()  [unwired: 1 in, 5 out]
        n518 = Enqueue Element(queue=w1096, element=Control_3."delete cycle") -> (queue out=w1095:refnum<queue>)  [unwired: 2 in, 2 out]
        n519 = Enqueue Element(queue=w1095, element=Control_3."update list 2") -> ()  [unwired: 2 in, 3 out]
      }
      event Value Change {
        n520 = event-data() -> ()  [unwired: 1 in, 5 out]
        n521 = Enqueue Element(queue=w1099, element=Control_3."Total time calc") -> ()  [unwired: 2 in, 3 out]
      }
      event "Cycle Pattern": Mouse Up; "Cycle Pattern": Value Change {
        n522 = event-data() -> ()  [unwired: 1 in, 3 out]
        n523 = property on="Cycle Pattern" class="Tbl (strict)"() -> ("EditPos"=w1106:T3)  [unwired: 2 in, 2 out]
        n524 = Unbundle By Name(w1106) -> ("Row"=w1103:i32, "Column"=w1108:i32)
        n525 = Less?(x=w1103, y=30) -> (x < y?=w1107:bool)
        n526 = case shown="True" w1107 {
          tunnel: w1108 -> [_ w1110]
          tunnel: w1104 -> [_ w1113]
          frame False {
            n527 = One Button Dialog(message="This table is limited to 30 entries!") -> ()  [unwired: 1 in, 1 out]
          }
          frame True {
            n528 = Equal?(x=w1110, y=1) -> (x = y?=w1114:bool)
            n529 = case shown="True" w1114 {
              tunnel: w1113 -> [w1117 w1120]
              tunnel: [w1116 w1119] -> w1112
              frame False {
                n530 = Enqueue Element(queue=w1117, element=Control_3."update Cycle pattern ") -> (queue out=w1116:refnum<queue>)  [unwired: 2 in, 2 out]
              }
              frame True {
                n531 = Enqueue Element(queue=w1120, element=Control_3."load cycle name") -> (queue out=w1119:refnum<queue>)  [unwired: 2 in, 2 out]
              }
            }
            n532 = Enqueue Element(queue=w1112, element=Control_3."Total time calc") -> ()  [unwired: 2 in, 3 out]
          }
        }
        "Flag 2" <- TRUE
      }
      event "Compile Test Button": Value Change {
        n533 = event-data() -> ()  [unwired: 1 in, 5 out]
        n534 = local read "Flag 2"() -> (w1122:bool)
        n535 = case shown="True" w1122 {
          tunnel: w1126 -> [w1127 w1131]
          tunnel: [w1127 w1128] -> w1124
          frame False {
          }
          frame True {
            n536 = Enqueue Element(queue=w1131, element=Control_3."save cycle") -> (queue out=w1129:refnum<queue>)  [unwired: 2 in, 2 out]
            n537 = Enqueue Element(queue=w1129, element=Control_3."update list 2") -> (queue out=w1128:refnum<queue>)  [unwired: 2 in, 2 out]
          }
        }
        n538 = Enqueue Element(queue=w1124, element=Control_3."load test array") -> ()  [unwired: 2 in, 3 out]
      }
      event Value Change {
        n539 = event-data() -> ()  [unwired: 1 in, 5 out]
        n540 = Enqueue Element(queue=w1134, element=Control_3."check scycle name") -> ()  [unwired: 2 in, 3 out]
      }
      event Value Change {
        n541 = event-data() -> ()  [unwired: 1 in, 5 out]
        n542 = Enqueue Element(queue=w1135, element=Control_3."check cycle name") -> ()  [unwired: 2 in, 3 out]
      }
      event Value Change {
        n543 = event-data() -> ()  [unwired: 1 in, 5 out]
        n544 = Square(x="Sample Diameter (mm)") -> (x^2=w1144:T1)
        n545 = Compound Arithmetic op=MULTIPLY(w1144, "Sample Length (mm)", "Number of Samples", 3.141592653589793) -> (w1143:T1)
        n546 = Divide(x=w1143, y=4000000.0) -> (x/y=→"Sample Volume (litres)":T1)
      }
      event Value Change {
        # "O2Eq"
        n547 = event-data() -> ()  [unwired: 1 in, 5 out]
        n548 = local write "Inlet LAMBDA"("Inlet LAMBDA") -> ()
        n549 = local write "Inlet O2 (%)"("Inlet O2 (%)") -> ()
        n550 = Decrement(x="Inlet LAMBDA") -> (x-1=w1159:T1)
        n551 = Multiply(x=4.76, y="Inlet LAMBDA") -> (x*y=w1155:T1)
        n552 = Multiply(x=w1159, y=100.0) -> (x*y=w1157:T1)
        n553 = Add(x=0.33, y=w1155) -> (x+y=w1153:T1)
        n554 = Divide(x=w1157, y=w1153) -> (x/y=w1152:T1)
        n555 = Subtract(x="Inlet O2 (%)", y=w1152) -> (x-y=w1150:T1)
        n556 = Multiply(x=w1150, y=2.0) -> (x*y=→"CO Theory (%)":T1)
        n557 = Divide(x=w1150, y=4.5) -> (x/y=→"HC Theory (%)":T1)
      }
      event Value Change {
        n558 = event-data() -> ()  [unwired: 1 in, 5 out]
        n559 = local write "NO ppm Loff"("NO ppm Loff") -> ()
        n560 = local write "NO:CO Ratio"("NO:CO Ratio") -> ()
        n561 = Divide(x="NO ppm Loff", y=T1 10000.0) -> (x/y=w1162:T1)
        n562 = Multiply(x="NO:CO Ratio", y=w1162) -> (x*y=→"CO Theory (%)":T1)
      }
      event Value Change {
        n563 = event-data() -> ()  [unwired: 1 in, 5 out]
        n564 = local read "Sample Volume (litres)"() -> (w1167:T7)
        n565 = Equal?(x=w1167, y=0.0) -> (x = y?=w1166:bool)
        n566 = case shown="False" w1166 {
          tunnel: w1167 -> [w1172 _]
          tunnel: "Test Flow Rate(g/s)" -> [w1169 _]
          frame False {
            w1174 = 60.0 ("y")
            n567 = Multiply(x=w1169, y=w1174) -> (x*y=w1176:T1)
            n568 = Divide(x=w1176, y=1.2) -> (x/y=w1171:T1)
            "Vol Flow @ STP (l/min)" <- w1171
            n569 = Multiply(x=w1171, y=w1174) -> (x*y=w1173:T1)
            n570 = Divide(x=w1173, y=w1172) -> (x/y=→"Space Velocity (h-1)":T1)
          }
          frame True {
            n571 = One Button Dialog(message="Review sample specification first!") -> ()  [unwired: 1 in, 1 out]
          }
        }
      }
      event "Execute Leak Test Button": Value Change {
        n572 = event-data() -> ()  [unwired: 1 in, 5 out]
        n573 = flat-sequence {
          tunnel: w1179 -> [w1182]
          tunnel: [w1182] -> w1178
          tunnel: w1178 -> [w1185]
          frame #0 {
            n574 = local write "Test number"(u16 5) -> ()
            n575 = local write "Enum 1"(u16 3 ("Test number")) -> ()
          }
          frame #1 {
            n576 = Enqueue Element(queue=w1185, element=Control_3."main" ("Enum")) -> (queue out=w1183:refnum<queue>)  [unwired: 2 in, 2 out]
            n577 = Enqueue Element(queue=w1183, element=Control_3."start test" ("Enum")) -> ()  [unwired: 2 in, 3 out]
          }
        }
      }
      event "Start Test Button": Value Change {
        # "Start Test Button - added function of if log button not pressed, pop up window generated to ask \"Currently no logging data, do you wish to continue\" If no test stops If yes test starts - Not Tested 141105 JS"
        n578 = event-data() -> ()  [unwired: 1 in, 5 out]
        n579 = flat-sequence {
          tunnel: w1188 -> [w1191]
          tunnel: [w1191] -> w1187
          tunnel: w1187 -> [w1193]
          frame #0 {
            n580 = local write "Enum 1"(u16 1 ("Test number")) -> ()
            "Test number" <- "Select Test Type"
          }
          frame #1 {
            n581 = local read "Log Test Button"() -> (w1192:bool)
            n582 = case shown="False" w1192 {
              tunnel: w1193 -> [w1194 w1202]
              frame False {
                n583 = Two Button Dialog(message="Currently not logging Test Data\nDo you wish to continue?") -> (T button?=w1196:bool)  [unwired: 2 in]
                n584 = case shown="True" w1196 {
                  tunnel: w1194 -> [_ w1198]
                  frame False {
                  }
                  frame True {
                    n585 = Enqueue Element(queue=w1198, element=Control_3."main" ("Enum")) -> (queue out=w1201:refnum<queue>)  [unwired: 2 in, 2 out]
                    n586 = property on="Stop Test Button" class="Bool"("DisabledEnum"=T13."Enabled" ("Disabled")) -> ()  [unwired: 2 in, 2 out]
                    n587 = Enqueue Element(queue=w1201, element=Control_3."start test" ("Enum")) -> ()  [unwired: 2 in, 3 out]
                  }
                }
              }
              frame True {
                n588 = Enqueue Element(queue=w1202, element=Control_3."main" ("Enum")) -> (queue out=w1206:refnum<queue>)  [unwired: 2 in, 2 out]
                n589 = property on="Stop Test Button" class="Bool"("DisabledEnum"=T13."Enabled" ("Disabled")) -> ()  [unwired: 2 in, 2 out]
                n590 = Enqueue Element(queue=w1206, element=Control_3."start test" ("Enum")) -> ()  [unwired: 2 in, 3 out]
              }
            }
          }
          frame #2 {
          }
        }
      }
      event "Stop Test Button": Value Change {
        # "Stop Test Button - Currently stops test and disconnects from MKS Analysers, need to remove MKS analysers and add to additional settings 141105 JS"
        n591 = event-data() -> ()  [unwired: 1 in, 5 out]
        n592 = flat-sequence {
          tunnel: w1212 -> [w1214]
          tunnel: [w1214] -> w1211
          tunnel: [w1213] -> w1209
          tunnel: w1211 -> [w1218]
          tunnel: [w1217] -> w1210
          tunnel: w1209 -> [w1217]
          tunnel: [w1216] -> w1208
          tunnel: w1210 -> [w1222]
          tunnel: w1208 -> [w1221]
          tunnel: [T13."Disabled and Grayed Out" ("Disabled")] -> w1207
          frame #0 {
            n593 = local read "Connected?"() -> (w1213:bool)
            n594 = local write "Stop Cmd"(T1 1.0 ("Stop Cmd")) -> ()
          }
          frame #1 {
            n595 = Enqueue Element(queue=w1218, element=Control_3."main" ("Enum")) -> (queue out=w1216:refnum<queue>)  [unwired: 2 in, 2 out]
          }
          frame #2 {
            n596 = case shown="True" w1222 {
              tunnel: w1221 -> [w1223 w1226]
              tunnel: [w1223 w1225] -> _
              frame False {
              }
              frame True {
                n597 = local write "Connected?"(FALSE ("Connected?")) -> ()
                n598 = Enqueue Element(queue=w1226, element=Control_3."Multigas disconnect" ("Enum")) -> (queue out=w1225:refnum<queue>)  [unwired: 2 in, 2 out]
              }
            }
          }
        }
        n599 = property on="Stop Test Button" class="Bool"("DisabledEnum"=w1207) -> ()  [unwired: 2 in, 2 out]
      }
      event "Stopped?": Value Change {
        n600 = event-data() -> ()  [unwired: 1 in, 5 out]
        n601 = flat-sequence {
          tunnel: w1230 -> [w1234]
          tunnel: [w1233] -> w1229
          tunnel: [w1232] -> w1228
          tunnel: w1229 -> [w1236]
          tunnel: w1228 -> [w1235]
          frame #0 {
            n602 = local read "Connected?"() -> (w1232:bool)
            n603 = Enqueue Element(queue=w1234, element=Control_3."main" ("Enum")) -> (queue out=w1233:refnum<queue>)  [unwired: 2 in, 2 out]
          }
          frame #1 {
            n604 = case shown="True" w1235 {
              tunnel: w1236 -> [_ w1237]
              frame False {
              }
              frame True {
                n605 = local write "Connected?"(FALSE ("Connected?")) -> ()
                n606 = Enqueue Element(queue=w1237, element=Control_3."Multigas disconnect" ("Enum")) -> ()  [unwired: 2 in, 3 out]
              }
            }
          }
        }
      }
      event "Alarm ack": Value Change {
        # "system alarm - set to off"
        n607 = event-data() -> ()  [unwired: 1 in, 5 out]
        n608 = local write "Acknowledge"(TRUE ("Acknowledge")) -> ()
        n609 = property on="Soft Alarm" class="Bool (strict)"("Value"=FALSE ("Acknowledge")) -> ()  [unwired: 2 in, 2 out]
        n610 = property on="Alarm ack" class="Bool"("DisabledEnum"=T13."Disabled and Grayed Out" ("Disabled")) -> ()  [unwired: 2 in, 2 out]
      }
      event "Purge System": Value Change {
        n611 = event-data() -> ()  [unwired: 1 in, 5 out]
        n612 = flat-sequence {
          tunnel: w1244 -> [w1246]
          tunnel: [w1246] -> w1243
          tunnel: w1243 -> [w1247]
          frame #0 {
            n613 = local write "Enum 1"(u16 4 ("Test number")) -> ()
          }
          frame #1 {
            n614 = Enqueue Element(queue=w1247, element=Control_3."start test" ("Enum")) -> ()  [unwired: 2 in, 3 out]
          }
        }
      }
      event "Clear log": Value Change {
        n615 = event-data() -> ()  [unwired: 1 in, 5 out]
        n616 = local write "Table"(string[][] [] ("Table")) -> ()
      }
      event "Advanced settings": Value Change {
        # "To be updated - To Include:\nFile Path\nAnalyser on/off switches\nRe-design of layout"
        # "SO2 conc\nNOx conc\nCO conc\nHC conc\nBleed ratio N2\nBleed ratio CO2"
        n617 = event-data() -> ()  [unwired: 1 in, 5 out]
        n618 = call "Advanced settings MAX.vi"() -> ("output cluster"=→"output cluster":T14)  [unwired: 1 in]
      }
    }
    "stop 2" <- w1025
  }
  n619 = local write "stop 2"(w9) -> ()
  n620 = node-c288(w6) -> ()  [unwired: 1 out]
  "Table" <- string[][] [] ("Table")
